vi "Vision_demo.vi"() -> ()   [LabVIEW 2011]
doc: "Use this template to build a standard state machine design pattern. Each state executes code and determines which state to transition to. Contrast this design pattern with the User Interface Event Handler pattern, in which code executes in response to user actions. Contrast this design pattern also with the Queued Message Handler pattern, in which each message handling code can queue zero or more new messages."
uses:
  StateMachineStates 1.ctl
  <vilib>/DAQmx/write.llb/DAQmx Write (Digital Bool 1Line 1Point).vi
  <vilib>/DAQmx/read.llb/DAQmx Read (Digital Bool 1Line 1Point).vi
  <vilib>/DAQmx/read.llb/DAQmx Read (Counter U32 1Chan 1Samp).vi
  <vilib>/DAQmx/miscellaneous.llb/DAQmx Fill In Error Info.vi
  <vilib>/DAQmx/create/channels.llb/DAQmx Create Channel (CI-Count Edges).vi
  <vilib>/DAQmx/read.llb/DAQmx Read (Counter DBL 1Chan 1Samp).vi
  <vilib>/DAQmx/create/channels.llb/DAQmx Create Channel (CI-Pulse Width).vi
panel:
  out "Set 4":bool[](array[boolean])
  out "Set 3":bool[](array[boolean])
  out "Set 2":bool[](array[boolean])
  out "Set 1":bool[](array[boolean])
  out "Photon time (ms)":dbl format="%.2f"
  in  "Interval (ms)":u32
  out "Repetition":dbl
  in  "Repetitions":dbl=1.0
  out "WP time (ms)":u32
  out "VISA Handle out":refnum<visa-resource-name>="ASRL5::INSTR"
  out "Initializing":bool
  out "Trial mode":T1(ring)
  in  "Frequency of LED trials\nfor Mixed mode":dbl=30.0
  out "Bright trial\nrequested":bool
  out "Observer Ready":bool
  in  "Bright/mixed mode \nLED voltage (V)":dbl=2.6 min=-3.0 max=4.0 format="%.2f"
  in  "Manual voltage (V)":dbl=2.6 format="%.2p"
  in  "GPIB address":string="15"
  in  "Period (ms)":i64=20
  in  "Pulse length (ms)":dbl=50.0
  out "L/R WP":dbl format="%.2f"
  in  "Manually \ninitialize":bool
  in  "COM for WPs":u8=5
  in  "L/R control method":enum16{"Liquid crystal", "Motorized waveplate"}(ring)=enum."Motorized waveplate"
  out "Blocked trial #":i32
  in  "Manual photon #":i32
  out "Photon #":i32
  out "LED Voltage":dbl
  in  "Blocking requirements":cluster{"Value":dbl, " Number":i32}[](array[cluster])
  in  "Manual":bool
  in  "Path":path=path "C:/Users/Lab/Dropbox/Vision software/Data"
  out "Counts 2":u32
  out "Counts 1":u32
  in  "Delay for APDs (ms)":u32=25
  in  "Counter 2":tag="Dev1/ctr1"
  in  "Counter 1":tag="Dev1/ctr0"
  out "Trial #":i32
  in  "Mode":T2(ring)=enum."Mixed"
  in  "Audio":bool=TRUE
  in  "Self-paced":bool
  out "Stimulus":bool
  out "Location Set":bool
  out "Stimulus \nlocation":string
  out "Waiting":bool
  out "Observer Responded":bool
  out "Response \ntime (ms)":dbl
  out "Observer \nchoice":string
  out "Confidence":i32
  in  "stop":bool
  in  "Next Trial":bool
  in  "Create New File":bool
  out "Subject #":string
  # "Settings for Blocking\nand Mixed Mode"
  # "Instructions: Run VI. Enter blocking requirements, then press\nCreate New File. Initialize waveplates if necessary, and set\nhighlighted controls to desired values. Press Next Trial to begin."
  # "Researcher Interface"
  # "Trial Options"
  # "Counter Options\n(same for LED &\ndetector tests)"
  # "Trial Information"
  # "Enter pre-set blocking \nrequirements\nbefore creating a new file."
  # "Troubleshooting"
  # "Photon Options"
  # "LED Options"
  # "Waveplates"
  # "Status"
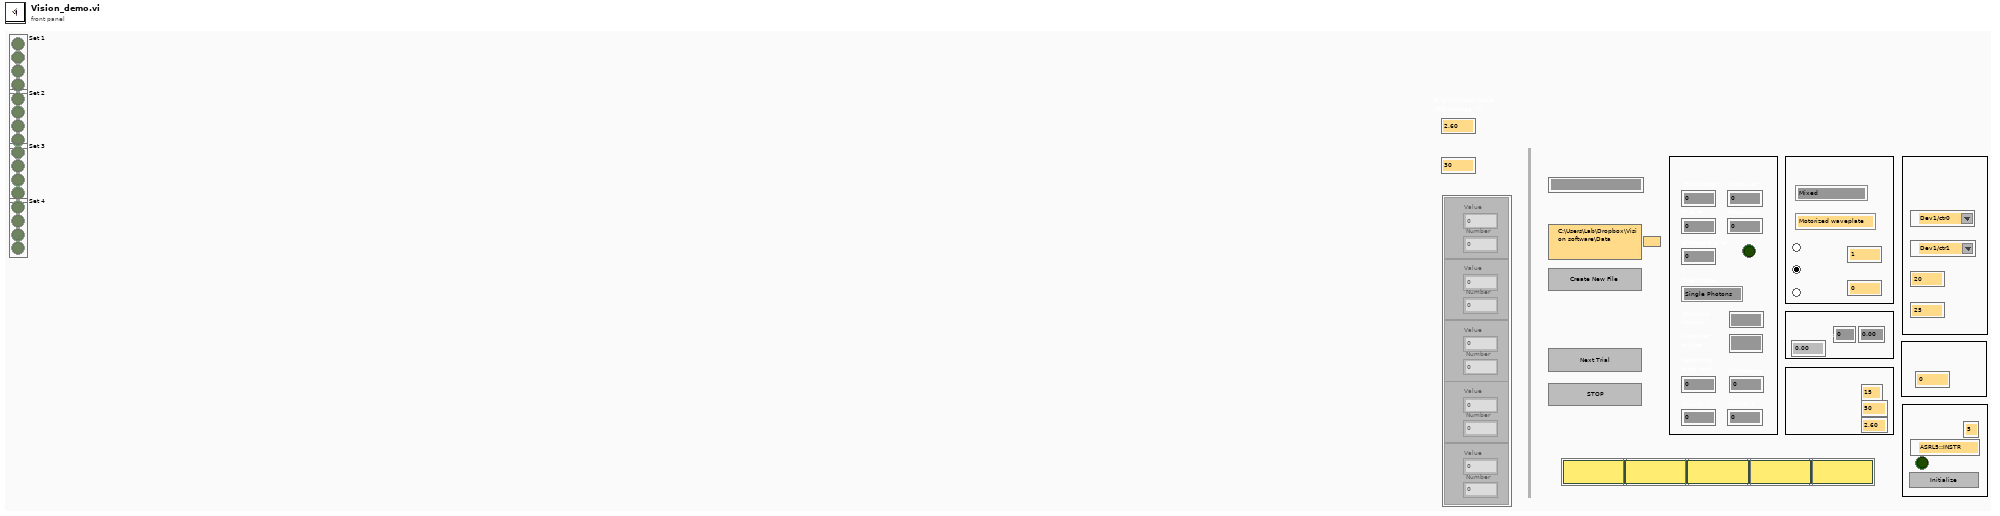
[diagram p1: front panel]
types:
  T1 = enum16{"Single Photons", "Detector Tests", "LED", "Mixed LED"}
  T2 = enum16{"Single Photons", "Detector Tests", "LED", "Mixed"}
  T3 = typedef "StateMachineStates 1.ctl" = enum16{"WaitResearcher", "SetWP", "SetLC", "WaitObserverReady", "Photons", "Detectors", "LED", "WaitObserverResponse", "CleanUp", "Stop"}
  T4 = enum16{"0", "1", "2", "3", "4", "5", "6", "7", "8", "9", "A", "B", "C", "D", "E", "F", "G", "H", "I", "J", "K", "L", "M", "N", "O", "P", "Q", "R", "S", "T", "U", "V", "W", "X", "Y", "Z", "F1", "F2", "F3", "F4", "F5", "F6", "F7", "F8", "F9", "F10", "F11", "F12", "F13", "F14", "F15", "ADD", "BACK", "BACKSLASH", "CAPITAL", "COMMA", "DECIMAL", "DELETE", "DIVIDE", "DOWN", "END", "EQUALS", "ESCAPE", "GRAVE (`)", "HOME", "INSERT", "LBRACKET", "LCONTROL", "LEFT", "L ALT", "LSHIFT", "LWIN", "MINUS", "MULTIPLY", "NEXT", "NUMLOCK", "NUMPAD_0", "NUMPAD_1", "NUMPAD_2", "NUMPAD_3", "NUMPAD_4", "NUMPAD_5", "NUMPAD_6", "NUMPAD_7", "NUMPAD_8", "NUMPAD_9", "PAUSE", "PERIOD", "PRIOR (PG UP)", "RBRACKET", "RCONTROL", "RETURN", "RIGHT", "R ALT", "RSHIFT", "RWIN", "SCROLL", "SEMICOLON", "SLASH", "SPACE", "SUBTRACT", "TAB", "UP", "ENTER (num pad)", "' (quote)"}
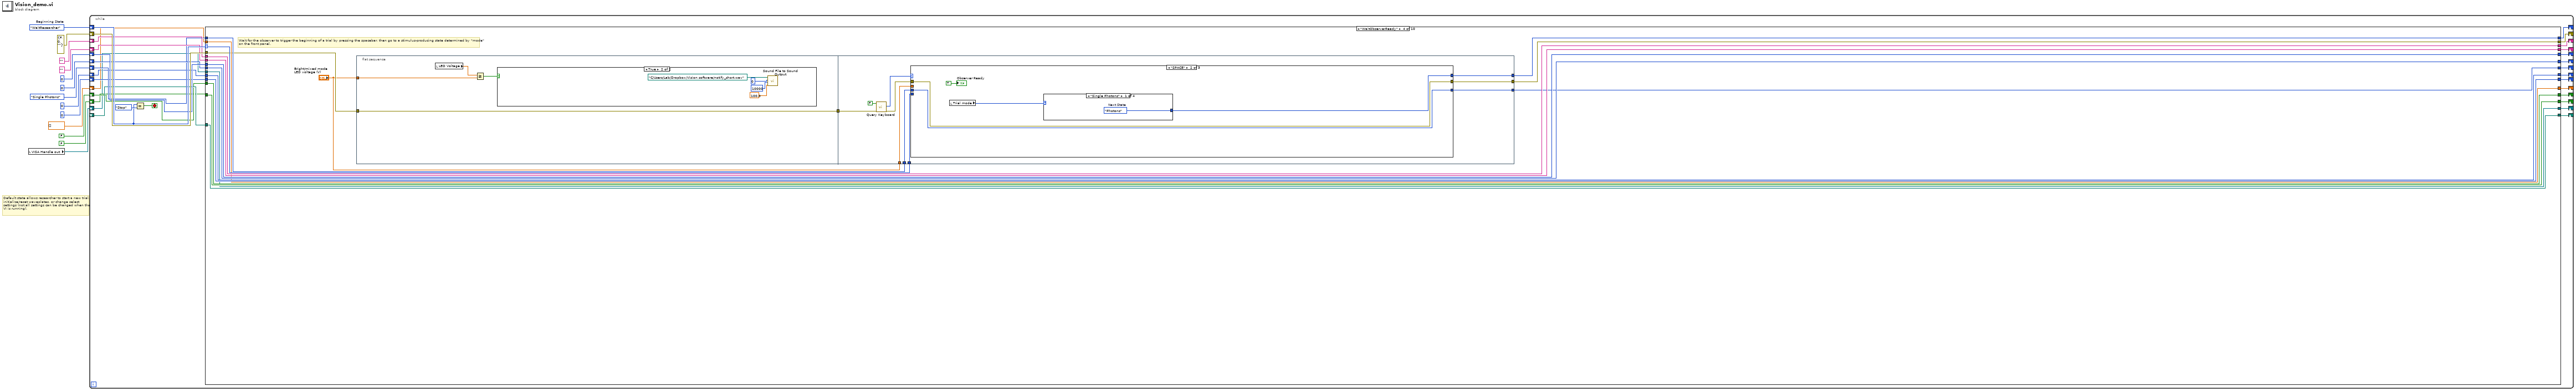
[diagram p0: block diagram]
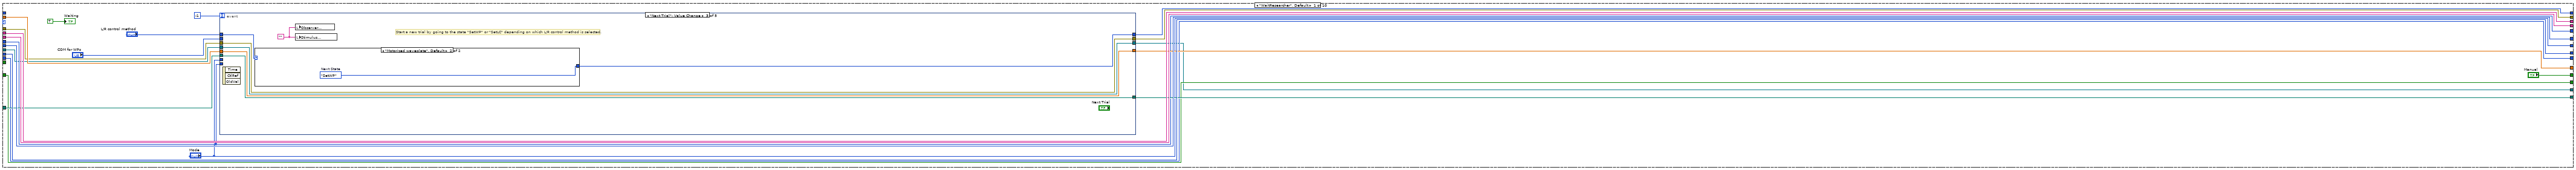
[diagram p2: hidden frame]
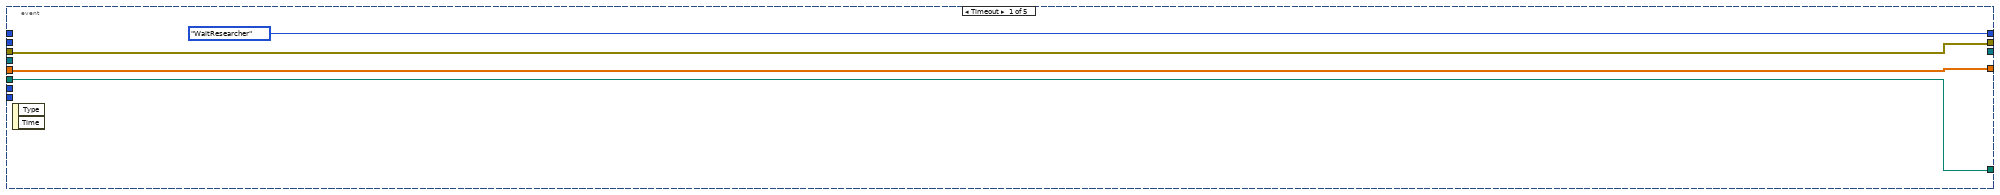
[diagram p3: hidden frame]
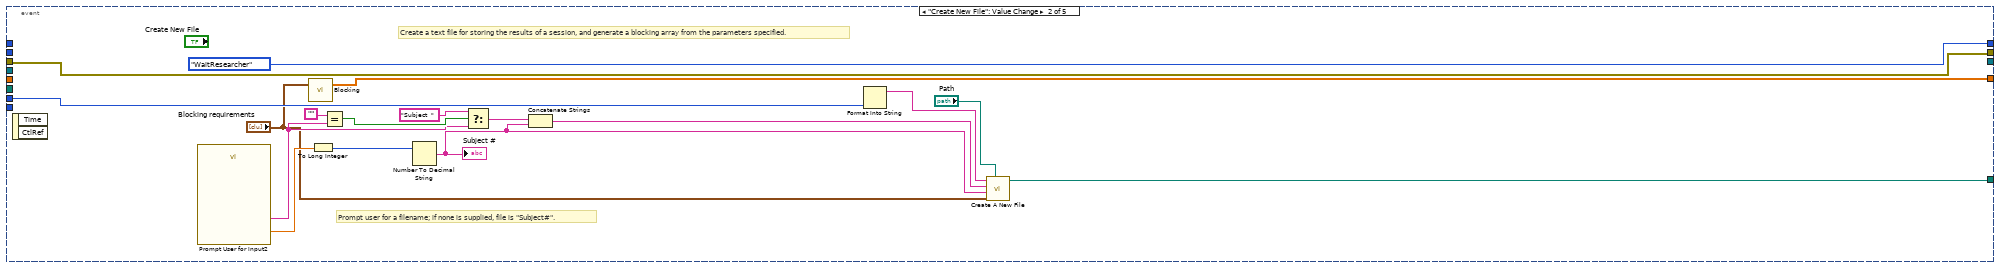
[diagram p4: hidden frame]
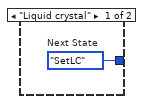
[diagram p5: hidden frame]
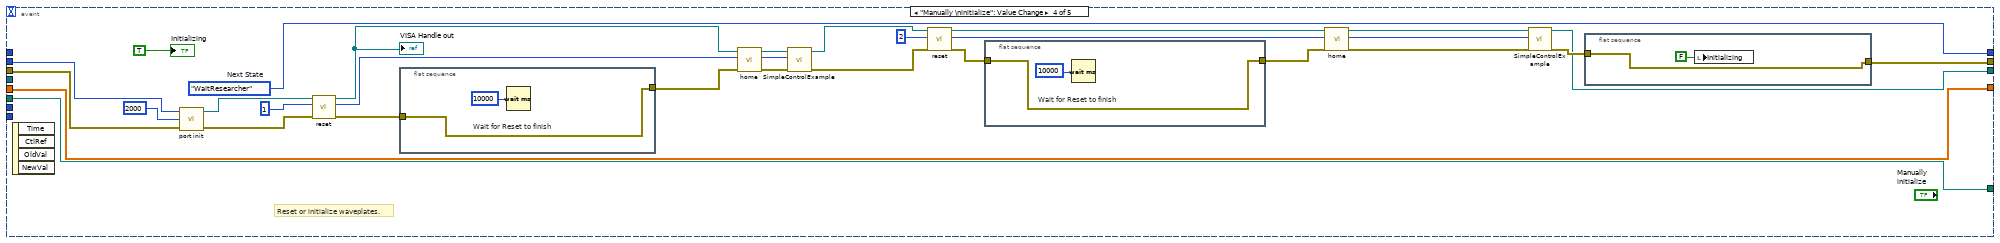
[diagram p6: hidden frame]
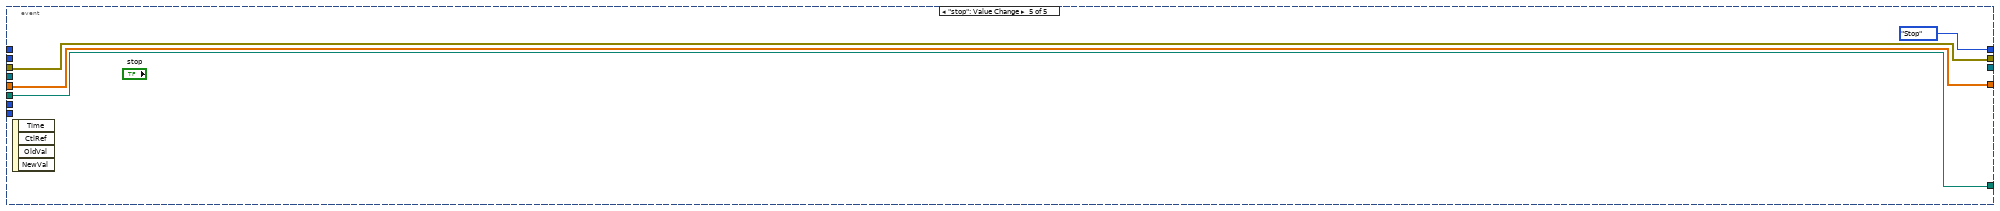
[diagram p7: hidden frame]
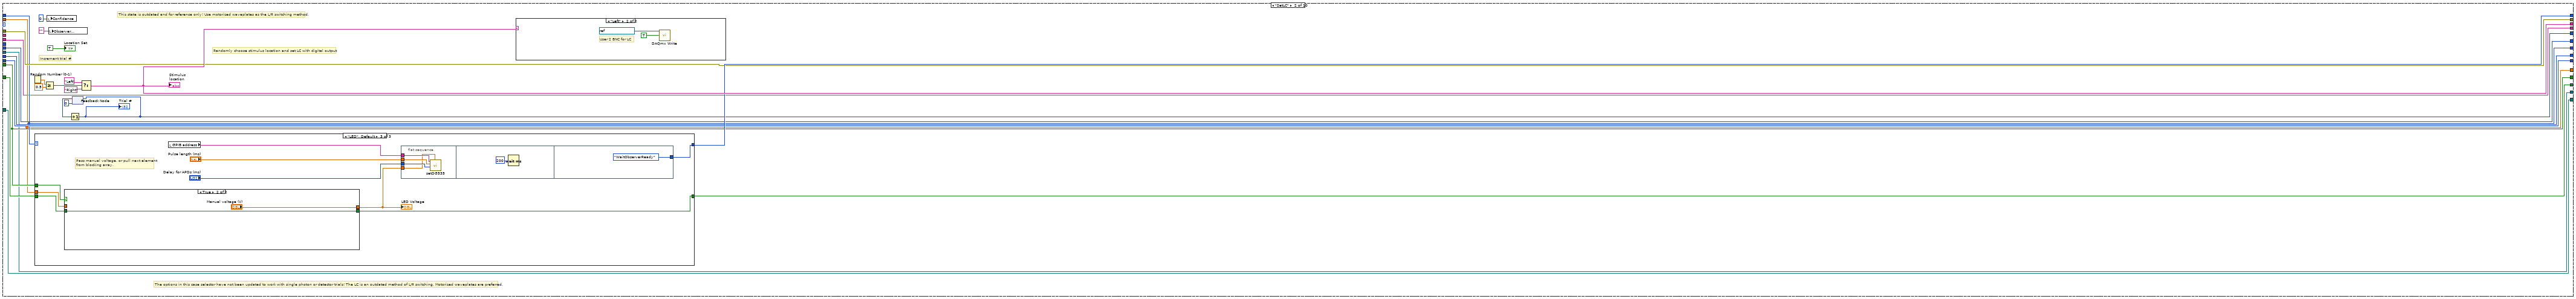
[diagram p8: hidden frame]
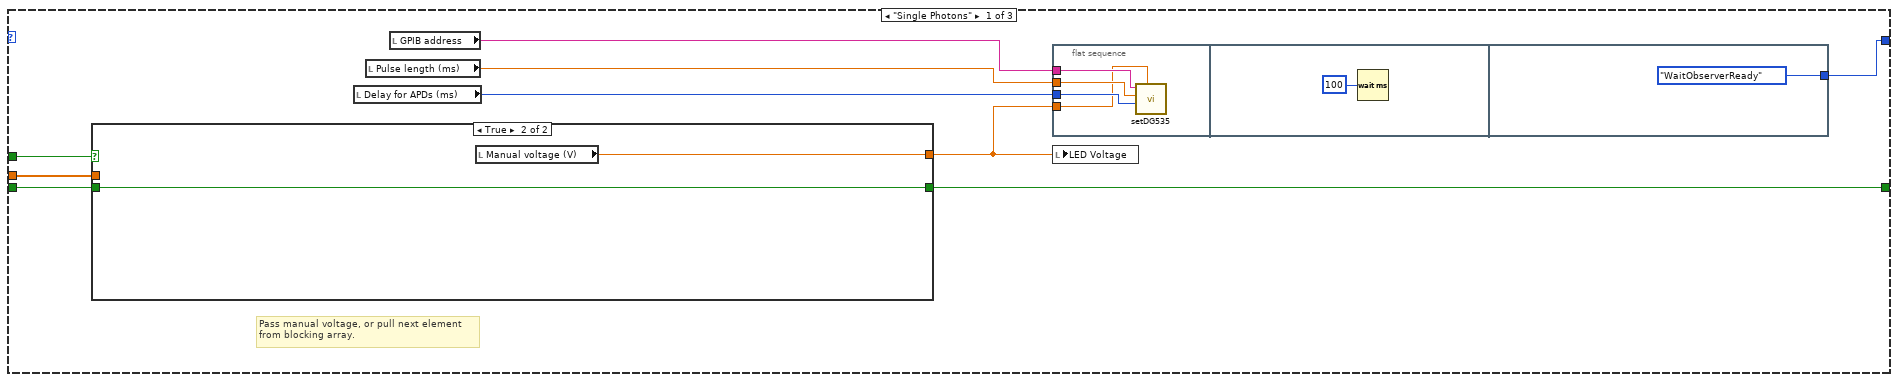
[diagram p9: hidden frame]
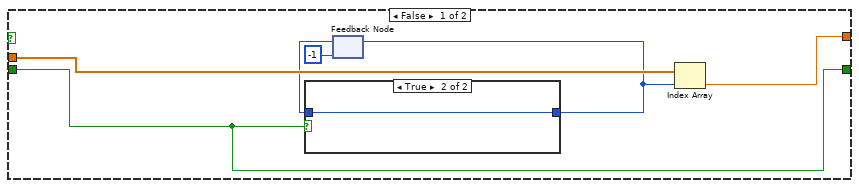
[diagram p10: hidden frame]
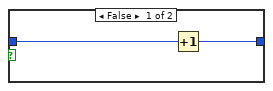
[diagram p11: hidden frame]
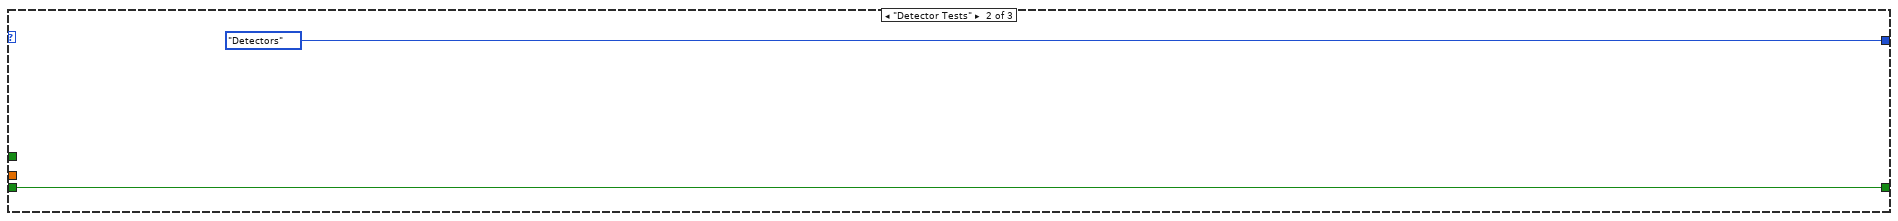
[diagram p12: hidden frame]
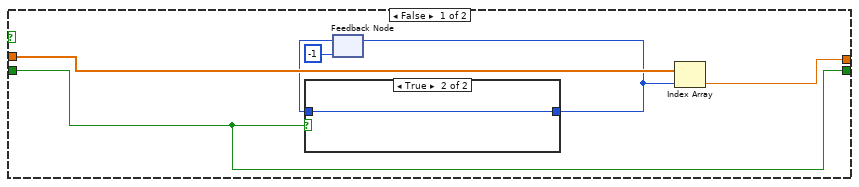
[diagram p13: hidden frame]
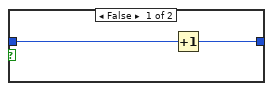
[diagram p14: hidden frame]
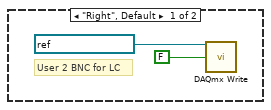
[diagram p15: hidden frame]
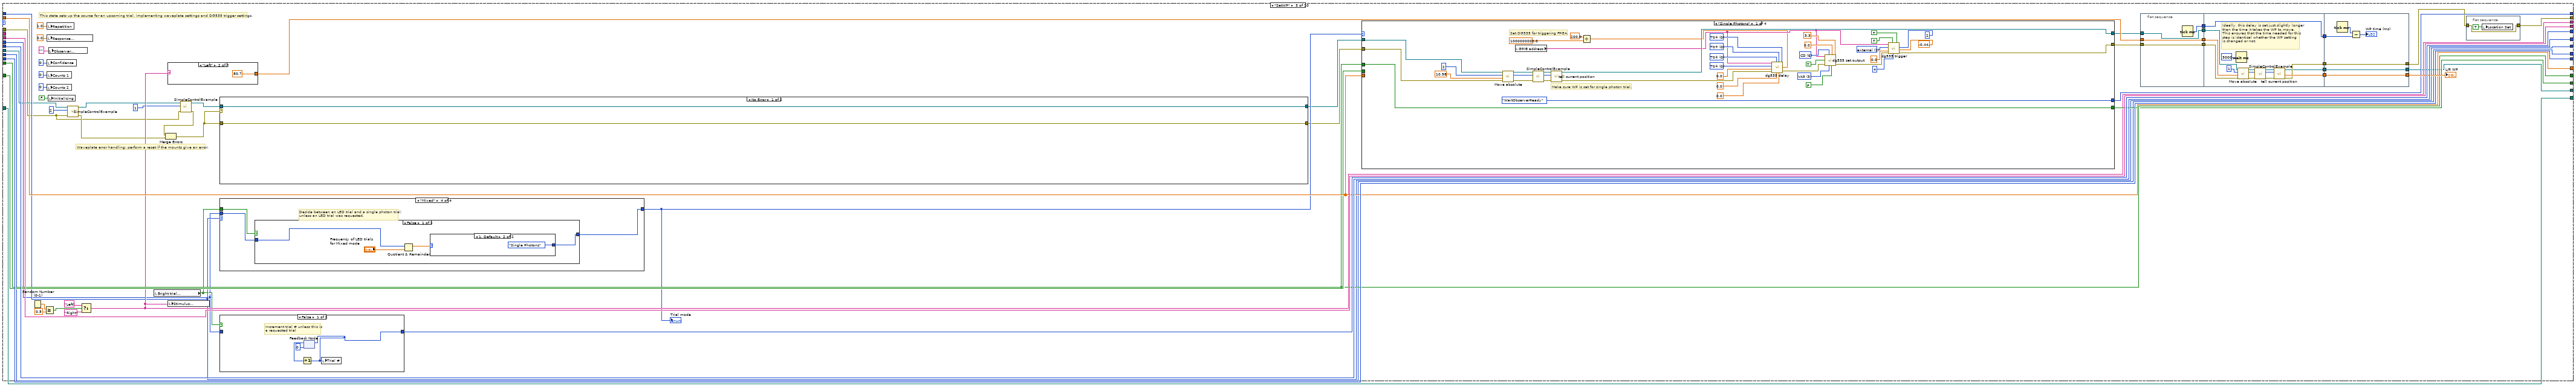
[diagram p16: hidden frame]
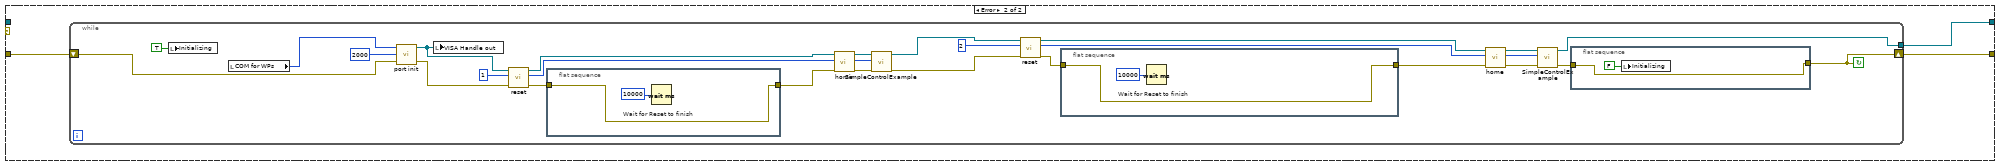
[diagram p17: hidden frame]
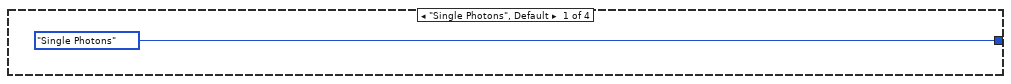
[diagram p19: hidden frame]
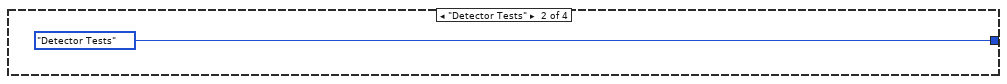
[diagram p20: hidden frame]
diagram:
  w13 = StateMachineStates_1."WaitResearcher"  # Beginning State
  # "Default state allows researcher to start a new trial,\ninitialize/reset waveplates, or change select\nsettings (not all settings can be changed when the\nVI is running)."
  n1 = local read "VISA Handle out"() -> (w1:refnum<visa-resource-name>)
  n2 = while {
    shift-right: [w40] -> _
    shift-left: w13 -> [w41]
    shift-right: [w19] -> _
    shift-left: errorcluster {"status"=FALSE, "code"=0, "source"=""} ("error out") -> [w39]
    shift-right: [w38] -> _
    shift-left: "" -> [w37]
    shift-right: [w36] -> _
    shift-left: "" ("Observer choice") -> [w35]
    shift-right: [w34] -> _
    shift-left: 0 -> [w33]
    shift-right: [w32] -> _
    shift-left: 0 ("Confidence") -> [w31]
    shift-right: [w30] -> _
    shift-left: T2."Single Photons" ("Mode") -> [w29]
    shift-right: [w28] -> _
    shift-left: u32 0 ("Counts 1") -> [w14]
    shift-right: [w27] -> _
    shift-left: u32 0 ("Counts 2") -> [w26]
    shift-right: [w25] -> _
    shift-left: _ -> [w24]
    shift-right: [w23] -> _
    shift-left: dbl[] [] ("Blocking array") -> [w22]
    shift-right: [w21] -> _
    shift-left: FALSE ("Manual") -> [w20]
    shift-right: [w18] -> _
    shift-left: FALSE ("Bright trial\nrequested") -> [w17]
    shift-right: [w16] -> _
    shift-left: w1 -> [w15]
    stop <- w43 stop-if-true
    n3 = Equal?(x=w41, y=StateMachineStates_1."Stop" ("States")) -> (x = y?=w43:bool)
    n4 = case shown="\"WaitObserverReady\"" w41 {
      selector: w41 -> [_ _ _ w521 _ _ _ _ _ _]
      tunnel: [w65 w154 w262 w522 StateMachineStates_1."WaitObserverResponse" ("Next State") w642 w832 w939 w1008 w1086] -> w40
      tunnel: [w50 w151 w261 w510 w601 w632 w818 w943 w991 w1091] -> w19
      tunnel: w39 -> [w51 w151 w220 w511 w587 w619 w834 w943 w985 w1090]
      tunnel: [w64 w155 w255 w525 w602 w645 w840 w945 w1004 w1102] -> w38
      tunnel: w37 -> [w64 _ _ w525 w602 w645 w840 w945 w1004 w1102]
      tunnel: [w63 w139 w272 w524 w605 w644 w813 w940 w1003 w1101] -> w36
      tunnel: w35 -> [w63 w139 w272 w524 w605 w644 _ _ w1003 w1101]
      tunnel: [w53 w145 w270 w523 w592 w635 w835 w944 w995 w1100] -> w34
      tunnel: w33 -> [w53 _ w236 w523 w592 w635 w835 w944 w995 w1100]
      tunnel: [w62 w152 w271 w520 w604 w643 w815 w938 w1007 w1099] -> w32
      tunnel: w31 -> [w62 w152 w271 w520 w604 w643 w815 _ w1007 w1099]
      tunnel: ["Mode" w144 w251 w518 w597 w641 w817 w937 w1002 w1098] -> w30
      tunnel: w29 -> [_ w144 w251 w517 w597 w641 w817 w937 w1002 w1098]
      tunnel: [w59 w148 w254 w516 w596 w640 w816 w936 w1000 w1097] -> w28
      tunnel: [w52 w147 w267 w515 w595 w639 w814 w935 w1001 w1096] -> w27
      tunnel: w14 -> [w59 w148 w254 w516 _ w640 _ w936 w1000 w1097]
      tunnel: w26 -> [w52 w147 w267 w515 _ w639 _ w935 w1001 w1096]
      tunnel: [w58 w146 w268 w514 w594 w638 w839 w934 w999 w1095] -> w25
      tunnel: w24 -> [w57 w146 w268 w514 w594 w638 w839 w934 w999 w1095]
      tunnel: [w56 w142 w266 w513 w593 w636 w836 w933 w997 w1094] -> w23
      tunnel: w22 -> [w55 w142 w266 w513 w593 w636 w836 w933 w997 w1094]
      tunnel: ["Manual" w143 w264 w512 w591 w637 w837 w932 w992 w1093] -> w21
      tunnel: w20 -> [_ w143 w264 w512 w591 w637 w837 w932 w989 w1093]
      tunnel: [w47 w140 w263 w508 w586 w633 w830 w931 w987 w1092] -> w18
      tunnel: w17 -> [w47 w141 w265 w508 w586 w633 w830 w931 _ w1092]
      tunnel: [w46 w136 w248 w507 w585 w634 w829 w930 w986 w1089] -> w16
      tunnel: w15 -> [w44 w136 w229 w507 w585 w634 w829 w930 w986 w1089]
      frame "WaitResearcher", Default {
        n5 = event shown="[2] \"Next Trial\": Value Change" {
          selector: _ -> [_ _ _ _ _]
          dyn-events: _ -> [_ _ _ _ _]
          timeout: -1 -> [_ _ _ _ _]
          tunnel: [StateMachineStates_1."WaitResearcher" ("Next State") StateMachineStates_1."WaitResearcher" ("Next State") w90 w125 StateMachineStates_1."Stop" ("Next State")] -> w65
          tunnel: "Mode" -> [_ w78 _ _ _]
          tunnel: [w69 w71 w92 w124 w134] -> w58
          tunnel: w57 -> [w69 _ w92 w124 w134]
          tunnel: [w68 w75 w91 w112 w133] -> w56
          tunnel: w55 -> [w68 _ w91 w112 w133]
          tunnel: w53 -> [_ _ _ _ _]
          tunnel: w51 -> [w67 w70 w88 w113 w132]
          tunnel: [w67 w70 w88 w102 w132] -> w50
          tunnel: "L/R control method" -> [_ _ w89 _ _]
          tunnel: "COM for WPs" -> [_ _ _ w100 _]
          tunnel: [_ _ w87 w98 _] -> w46
          tunnel: w44 -> [_ _ w87 _ _]
          event Timeout {
            n6 = event-data() -> ()  [unwired: 1 in, 2 out]
          }
          event "Create New File": Value Change {
            # "Create a text file for storing the results of a session, and generate a blocking array from the parameters specified."
            # "Prompt user for a filename; if none is supplied, file is \"Subject#\"."
            n7 = event-data() -> ()  [unwired: 1 in, 2 out]
            n8 = call "Prompt User for Input2"() -> ("Subject #"=w84:dbl, "Filename"=w81:string)  [unwired: 16 in, 2 out]
            n9 = call "Blocking.vi"("Blocking requirements"="Blocking requirements") -> ("Blocking array"=w75:dbl[])  [unwired: 2 in]
            n10 = To Long Integer(number=w84) -> (32bit integer=w85:i32)
            n11 = Equal?(x="", y=w81) -> (x = y?=w82:bool)
            n12 = Number To Decimal String(number=w85) -> (decimal integer string=w79:string)  [unwired: 1 in]
            "Subject #" <- w79
            n13 = Select(t="Subject  ", s=w82, f=w81) -> (s? t:f=w76:string)
            n14 = Concatenate Strings(w76, w79) -> (w72:string)
            n15 = Format Into String(w78) -> (resulting string=w77:string)  [unwired: 3 in, 1 out]
            n16 = call "Create A New File.vi"("Path in"="Path", "Blocking requirements"="Blocking requirements", "Subject #"=w79, "Filename"=w72, "Mode"=w77) -> ("Path out"=w71:path)  [unwired: 6 in]
          }
          event "Next Trial": Value Change {
            w93 = ""
            # "Start a new trial by going to the state \"SetWP\" or \"SetLC\" depending on which L/R control method is selected."
            n17 = event-data() -> ()  [unwired: 1 in, 3 out]
            n18 = case shown="\"Motorized waveplate\", Default" w89 {
              tunnel: [w94 w95] -> w90
              frame "Liquid crystal" {
                w94 = StateMachineStates_1."SetLC"  # Next State
              }
              frame "Motorized waveplate", Default {
                w95 = StateMachineStates_1."SetWP"  # Next State
              }
            }
            n19 = local write "Observer \nchoice"(w93) -> ()
            n20 = local write "Stimulus \nlocation"(w93) -> ()
          }
          event "Manually \ninitialize": Value Change {
            w125 = StateMachineStates_1."WaitResearcher"  # Next State
            # "Reset or initialize waveplates."
            n21 = event-data() -> ()  [unwired: 1 in, 4 out]
            n22 = call "port init.vi"("error in"=w113, "Timeout (300 ms)"=u32 2000, "SerialPort (1)"=w100) -> ("error out"=w120:errorcluster, "Visa Handle"=w119:refnum<visa-resource-name>)  [unwired: 1 in]
            n23 = call "reset.vi"("error in"=w120, "Axis in"=1, "VISA Handle in"=w119) -> ("error out"=w117:errorcluster, "Axis out"=w118:i32, "VISA Handle out"=w96:refnum<visa-resource-name>)  [unwired: 3 in, 1 out]
            "VISA Handle out" <- w96
            n24 = flat-sequence {
              tunnel: [w130] -> w116
              tunnel: w117 -> [w130]
              frame #0 {
                # "Wait for Reset to finish"
                n25 = Wait (ms)(milliseconds to wait=u32 10000) -> ()  [unwired: 1 out]
              }
            }
            n26 = call "home.vi"("error in"=w116, "Axis in"=w118, "VISA Handle in"=w96) -> ("error out"=w122:errorcluster, "Axis out"=w121:i32, "VISA Handle out"=w123:refnum<visa-resource-name>)  [unwired: 3 in, 1 out]
            n27 = call "SimpleControlExample.vi"("error in"=w122, "Axis in"=w121, "VISA Handle in"=w123) -> ("error out"=w101:errorcluster, "VISA Handle out"=w99:refnum<visa-resource-name>)  [unwired: 3 in, 2 out]
            n28 = call "reset.vi"("error in"=w101, "Axis in"=2, "VISA Handle in"=w99) -> ("error out"=w107:errorcluster, "Axis out"=w108:i32, "VISA Handle out"=w104:refnum<visa-resource-name>)  [unwired: 3 in, 1 out]
            n29 = flat-sequence {
              tunnel: [w128] -> w106
              tunnel: w107 -> [w128]
              frame #0 {
                # "Wait for Reset to finish"
                n30 = Wait (ms)(milliseconds to wait=u32 10000) -> ()  [unwired: 1 out]
              }
            }
            n31 = call "home.vi"("error in"=w106, "Axis in"=w108, "VISA Handle in"=w104) -> ("error out"=w110:errorcluster, "Axis out"=w109:i32, "VISA Handle out"=w111:refnum<visa-resource-name>)  [unwired: 3 in, 1 out]
            n32 = call "SimpleControlExample.vi"("error in"=w110, "Axis in"=w109, "VISA Handle in"=w111) -> ("error out"=w103:errorcluster, "VISA Handle out"=w98:refnum<visa-resource-name>)  [unwired: 3 in, 2 out]
            n33 = flat-sequence {
              tunnel: w103 -> [w127]
              tunnel: [w127] -> w102
              frame #0 {
                n34 = local write "Initializing"(FALSE ("Initializing waveplates")) -> ()
              }
            }
            "Initializing" <- TRUE ("Initializing waveplates")
          }
          event "stop": Value Change {
            n35 = event-data() -> ()  [unwired: 1 in, 4 out]
          }
        }
        "Waiting" <- TRUE ("Waiting")
      }
      frame "SetLC" {
        # "This state is outdated and for reference only! Use motorized waveplates as the L/R switching method."
        # "The options in this case selector have not been updated to work with single photon or detector trials! The LC is an outdated method of L/R switching. Motorized waveplates are preferred."
        # "Randomly choose stimulus location and set LC with digital output"
        # "Increment trial #"
        n36 = Random Number (0-1)() -> (number: 0 to 1=w160:dbl)
        n37 = case shown="\"LED\", Default" w144 {
          tunnel: [w166 StateMachineStates_1."Detectors" ("Next State") w191] -> w154
          tunnel: w143 -> [w169 _ w197]
          tunnel: w142 -> [w168 _ w196]
          tunnel: w141 -> [w165 w187 w190]
          tunnel: [w164 w187 w189] -> w140
          frame "Single Photons" {
            # "Pass manual voltage, or pull next element\nfrom blocking array."
            n38 = case shown="True" w169 {
              tunnel: [w180 w185] -> w161
              tunnel: w168 -> [w181 _]
              tunnel: w165 -> [w176 w186]
              tunnel: [w176 w186] -> w164
              frame False {
                n39 = feedback #1(-1 ("x+1")) -> (w179:i32)
                n40 = case shown="True" w176 {
                  tunnel: w179 -> [w183 w184]
                  tunnel: [w182 w184] -> w177
                  frame False {
                    n41 = Increment(x=w183) -> (x+1=w182:i32)
                  }
                  frame True {
                  }
                }
                n42 = feedback-in #1(w177) -> ()
                n43 = Index Array(array=w181, index=w177) -> (element=w180:dbl)
              }
              frame True {
                n44 = local read "Manual voltage (V)"() -> (w185:dbl)
              }
            }
            n45 = local read "Delay for APDs (ms)"() -> (w163:u32)
            n46 = local read "Pulse length (ms)"() -> (w162:dbl)
            n47 = local read "GPIB address"() -> (w167:string)
            n48 = flat-sequence {
              tunnel: w163 -> [w173]
              tunnel: w167 -> [w172]
              tunnel: w162 -> [w171]
              tunnel: w161 -> [w170]
              tunnel: [StateMachineStates_1."WaitObserverReady" ("Next State")] -> w166
              frame #0 {
                n49 = call "setDG535.vi"("amplitude"=w170, "Delay (ms)"=w173, "Pulse length (ms)"=w171, "GPIB address"=w172) -> ()  [unwired: 7 in, 1 out]
              }
              frame #1 {
                n50 = Wait (ms)(milliseconds to wait=u32 100) -> ()  [unwired: 1 out]
              }
              frame #2 {
              }
            }
            n51 = local write "LED Voltage"(w161) -> ()
          }
          frame "Detector Tests" {
          }
          frame "LED", Default {
            # "Pass manual voltage, or pull next element\nfrom blocking array."
            n52 = case shown="True" w197 {
              tunnel: [w208 "Manual voltage (V)"] -> w192
              tunnel: w196 -> [w209 _]
              tunnel: w190 -> [w204 w213]
              tunnel: [w204 w213] -> w189
              frame False {
                n53 = feedback #2(-1 ("x+1")) -> (w207:i32)
                n54 = case shown="True" w204 {
                  tunnel: w207 -> [w211 w212]
                  tunnel: [w210 w212] -> w205
                  frame False {
                    n55 = Increment(x=w211) -> (x+1=w210:i32)
                  }
                  frame True {
                  }
                }
                n56 = feedback-in #2(w205) -> ()
                n57 = Index Array(array=w209, index=w205) -> (element=w208:dbl)
              }
              frame True {
              }
            }
            "LED Voltage" <- w192
            n58 = local read "GPIB address"() -> (w194:string)
            n59 = flat-sequence {
              tunnel: "Delay for APDs (ms)" -> [w201]
              tunnel: w194 -> [w200]
              tunnel: "Pulse length (ms)" -> [w199]
              tunnel: w192 -> [w198]
              tunnel: [StateMachineStates_1."WaitObserverReady" ("Next State")] -> w191
              frame #0 {
                n60 = call "setDG535.vi"("amplitude"=w198, "Delay (ms)"=w201, "Pulse length (ms)"=w199, "GPIB address"=w200) -> ()  [unwired: 7 in, 1 out]
              }
              frame #1 {
                n61 = Wait (ms)(milliseconds to wait=u32 200) -> ()  [unwired: 1 out]
              }
              frame #2 {
              }
            }
          }
        }
        n62 = Greater Or Equal?(x=w160, y=0.5) -> (x >= y?=w158:bool)
        n63 = local write "Confidence"(0 ("Confidence")) -> ()
        n64 = local write "Observer \nchoice"("" ("Observer choice")) -> ()
        n65 = feedback #3(0 ("x+1")) -> (w150:i32)
        n66 = Increment(x=w150) -> (x+1=w145:i32)
        "Trial #" <- w145
        n67 = feedback-in #3(w145) -> ()
        n68 = Select(t="Left", s=w158, f="Right") -> (s? t:f=w155:string)
        "Stimulus \nlocation" <- w155
        n69 = case shown="\"Left\"" w155 {
          frame "Right", Default {
            # "User 2 BNC for LC"
            n70 = call-poly <vilib>:"DAQmx Write.vi"("task/channels in"=refnum<k21> "LC_Controller", "data"=FALSE) -> ()  [unwired: 11 in, 3 out]
          }
          frame "Left" {
            # "User 2 BNC for LC"
            n71 = call-poly <vilib>:"DAQmx Write.vi"("task/channels in"=refnum<k21> "LC_Controller", "data"=TRUE) -> ()  [unwired: 11 in, 3 out]
          }
        }
        "Location Set" <- TRUE ("LC Set")
      }
      frame "SetWP" {
        # "Waveplate error handling: perform a reset if the mounts give an error."
        # "This state sets up the source for an upcoming trial, implementing waveplate settings and DG535 trigger settings."
        n72 = Random Number (0-1)() -> (number: 0 to 1=w256:dbl)
        n73 = Greater Or Equal?(x=w256, y=0.5) -> (x >= y?=w258:bool)
        n74 = local write "Repetition"(1.0 ("Repitition #")) -> ()
        n75 = local write "Response \ntime (ms)"(0.0 ("Response \ntime (ms)")) -> ()
        n76 = local write "Confidence"(0 ("Confidence")) -> ()
        n77 = local write "Counts 1"(u32 0 ("Counts 1")) -> ()
        n78 = local write "Counts 2"(u32 0 ("Counts 2")) -> ()
        n79 = local write "Initializing"(FALSE ("Initializing waveplates")) -> ()
        n80 = local write "Observer \nchoice"("" ("Observer \nchoice")) -> ()
        n81 = call "SimpleControlExample.vi"("error in"=w220, "Axis in"=2, "VISA Handle in"=w229) -> ("error out"=w221:errorcluster, "VISA Handle out"=w227:refnum<visa-resource-name>)  [unwired: 3 in, 2 out]
        n82 = Select(t="Left", s=w258, f="Right") -> (s? t:f=w255:string)
        n83 = local read "Bright trial\nrequested"() -> (w237:bool)
        n84 = case shown="\"Left\"" w255 {
          tunnel: [35.7 ("New target position (units)") 80.7 ("New target position (units)")] -> w252
          frame "Right", Default {
          }
          frame "Left" {
          }
        }
        n85 = local write "Stimulus \nlocation"(w255) -> ()
        n86 = call "SimpleControlExample.vi"("error in"=w220, "Axis in"=1, "VISA Handle in"=w227) -> ("error out"=w222:errorcluster, "VISA Handle out"=w225:refnum<visa-resource-name>)  [unwired: 3 in, 2 out]
        n87 = Merge Errors(w222, w221) -> (w219:errorcluster)
        n88 = case shown="No Error" w219 {
          tunnel: w219 -> [w274 w277]
          tunnel: [w274 w275] -> w223
          tunnel: [w273 w276] -> w224
          tunnel: w225 -> [w273 _]
          frame No Error {
          }
          frame Error {
            n89 = while {
              tunnel: [w280] -> w276
              shift-right: [w278] -> w275
              shift-left: w277 -> [w283]
              stop <- w278 continue-if-true
              n90 = local write "Initializing"(TRUE ("Initializing waveplates")) -> ()
              n91 = local read "COM for WPs"() -> (w282:u8)
              n92 = call "port init.vi"("error in"=w283, "Timeout (300 ms)"=u32 2000, "SerialPort (1)"=w282) -> ("error out"=w301:errorcluster, "Visa Handle"=w281:refnum<visa-resource-name>)  [unwired: 1 in]
              n93 = local write "VISA Handle out"(w281) -> ()
              n94 = call "reset.vi"("error in"=w301, "Axis in"=1, "VISA Handle in"=w281) -> ("error out"=w299:errorcluster, "Axis out"=w300:i32, "VISA Handle out"=w284:refnum<visa-resource-name>)  [unwired: 3 in, 1 out]
              n95 = flat-sequence {
                tunnel: [w309] -> w298
                tunnel: w299 -> [w309]
                frame #0 {
                  # "Wait for Reset to finish"
                  n96 = Wait (ms)(milliseconds to wait=u32 10000) -> ()  [unwired: 1 out]
                }
              }
              n97 = call "home.vi"("error in"=w298, "Axis in"=w300, "VISA Handle in"=w284) -> ("error out"=w303:errorcluster, "Axis out"=w302:i32, "VISA Handle out"=w304:refnum<visa-resource-name>)  [unwired: 3 in, 1 out]
              n98 = call "SimpleControlExample.vi"("error in"=w303, "Axis in"=w302, "VISA Handle in"=w304) -> ("error out"=w286:errorcluster, "VISA Handle out"=w285:refnum<visa-resource-name>)  [unwired: 3 in, 2 out]
              n99 = call "reset.vi"("error in"=w286, "Axis in"=2, "VISA Handle in"=w285) -> ("error out"=w291:errorcluster, "Axis out"=w292:i32, "VISA Handle out"=w288:refnum<visa-resource-name>)  [unwired: 3 in, 1 out]
              n100 = flat-sequence {
                tunnel: [w307] -> w290
                tunnel: w291 -> [w307]
                frame #0 {
                  # "Wait for Reset to finish"
                  n101 = Wait (ms)(milliseconds to wait=u32 10000) -> ()  [unwired: 1 out]
                }
              }
              n102 = call "home.vi"("error in"=w290, "Axis in"=w292, "VISA Handle in"=w288) -> ("error out"=w294:errorcluster, "Axis out"=w293:i32, "VISA Handle out"=w295:refnum<visa-resource-name>)  [unwired: 3 in, 1 out]
              n103 = call "SimpleControlExample.vi"("error in"=w294, "Axis in"=w293, "VISA Handle in"=w295) -> ("error out"=w287:errorcluster, "VISA Handle out"=w280:refnum<visa-resource-name>)  [unwired: 3 in, 2 out]
              n104 = flat-sequence {
                tunnel: w287 -> [w306]
                tunnel: [w306] -> w278
                frame #0 {
                  n105 = local write "Initializing"(FALSE ("Initializing waveplates")) -> ()
                }
              }
            }
          }
        }
        n106 = case shown="\"Mixed\"" w251 {
          tunnel: [T1."Single Photons" ("Mode") T1."Detector Tests" ("Mode") T1."LED" ("Mode") w319] -> w250
          tunnel: w236 -> [_ _ _ w320]
          tunnel: w237 -> [_ _ _ w318]
          frame "Single Photons", Default {
          }
          frame "Detector Tests" {
          }
          frame "LED" {
          }
          frame "Mixed" {
            # "Decide between an LED trial and a single photon trial,\nunless an LED trial was requested."
            n107 = case shown="False" w318 {
              tunnel: w320 -> [w324 _]
              tunnel: [w321 T1."Mixed LED" ("Mode")] -> w319
              frame False {
                n108 = Quotient & Remainder(x=w324, y="Frequency of LED trials\nfor Mixed mode") -> (x-y*floor(x/y)=w322:dbl)  [unwired: 1 out]
                n109 = case shown="1, Default" w322 {
                  tunnel: [T1."Mixed LED" ("Mode") T1."Single Photons" ("Mode")] -> w321
                  frame 0 {
                  }
                  frame 1, Default {
                  }
                }
              }
              frame True {
              }
            }
          }
        }
        "Trial mode" <- w250
        n110 = case shown="False" w237 {
          tunnel: [w311 w314] -> w270
          tunnel: w236 -> [_ w314]
          frame False {
            # "Increment trial # unless this is\na requested trial"
            n111 = feedback #4(0 ("x+1")) -> (w313:i32)
            n112 = Increment(x=w313) -> (x+1=w311:i32)
            n113 = feedback-in #4(w311) -> ()
            n114 = local write "Trial #"(w311) -> ()
          }
          frame True {
          }
        }
        n115 = case shown="\"Single Photons\"" w250 {
          tunnel: [StateMachineStates_1."WaitObserverReady" ("Next State") StateMachineStates_1."Detectors" ("Next State") w456 w496] -> w262
          tunnel: w264 -> [w397 _ w459 _]
          tunnel: w266 -> [_ _ w458 _]
          tunnel: w265 -> [_ w437 w455 w482]
          tunnel: [w397 w437 w454 w482] -> w263
          tunnel: w223 -> [w388 w429 w443 w486]
          tunnel: [w358 w398 w442 w477] -> w246
          tunnel: w224 -> [w357 w427 w440 w484]
          tunnel: [w386 w426 w439 w483] -> w247
          frame "Single Photons" {
            w374 = u32 1 items=["internal", "external", "single shot", "burst", "line"] ("trigger")
            w376 = 3 items=["TTL", "NIM", "ECL", "VAR"] ("mode")
            w378 = u16 6 items=["T0", "A", "B", "AB", "C", "D", "CD"] ("output")
            w381 = u32 0 items=["T0+", "A+", "B+", "C+"] ("D=")
            w382 = u32 0 items=["T0+", "A+", "B+", "D+"] ("C=")
            w383 = u32 0 items=["T0+", "A+", "C+", "D+"] ("B=")
            w384 = u32 0 items=["T0+", "B+", "C+", "D+"] ("A=")
            # "Set DG535 for triggering FPGA."
            # "Make sure WP is set for single photon trial."
            n116 = call <instrlib>:"Move absolute.vi"("error in"=w388, "New target position (units)"=10.98, "Axis in"=2, "VISA Handle in"=w357) -> ("error out"=w390:errorcluster, "Axis out"=w391:i32, "VISA Handle out"=w392:refnum<visa-resource-name>)  [unwired: 2 in, 1 out]
            n117 = local read "GPIB address"() -> (w366:string)
            n118 = call "SimpleControlExample.vi"("error in"=w390, "Axis in"=w391, "VISA Handle in"=w392) -> ("error out"=w393:errorcluster, "Axis out"=w394:i32, "VISA Handle out"=w395:refnum<visa-resource-name>)  [unwired: 3 in, 1 out]
            n119 = call "tell current position.vi"("error in"=w393, "Axis in"=w394, "VISA Handle in"=w395) -> ("error out"=w359:errorcluster, "VISA Handle out"=w386:refnum<visa-resource-name>)  [unwired: 2 in, 3 out]
            n120 = Divide(x=200.0 ("D"), y=1000000000.0) -> (x/y=w360:dbl)
            n121 = call "dg535 delay.vi"("C"=0.0, "D"=w360, "D="=w381, "C="=w382, "B"=0.0 ("C"), "error in"=w359, "A"=0.0 ("D"), "B="=w383, "A="=w384, "GPIB address"=w366) -> ("error out"=w380:errorcluster)
            n122 = call "dg535 set output.vi"("GPIB address"=w366, "output"=w378, "set"=TRUE, "error in"=w380, "mode"=w376, "offset"=0.0, "amplitude"=3.3, "load"=FALSE) -> ("error out"=w367:errorcluster)  [unwired: 1 in]
            n123 = call "dg535 trigger.vi"("external trigger level"=sgl -0.45, "burst count"=2, "trigger slope"=TRUE, "burst period"=4, "input impedance"=TRUE, "error in"=w367, "internal/burst trigger rate"=0.0, "trigger"=w374, "GPIB address"=w366) -> ("error out"=w358:errorcluster)
          }
          frame "Detector Tests" {
            w414 = u32 1 items=["internal", "external", "single shot", "burst", "line"] ("trigger")
            w416 = 3 items=["TTL", "NIM", "ECL", "VAR"] ("mode")
            w418 = u16 6 items=["T0", "A", "B", "AB", "C", "D", "CD"] ("output")
            w421 = u32 0 items=["T0+", "A+", "B+", "C+"] ("D=")
            w422 = u32 0 items=["T0+", "A+", "B+", "D+"] ("C=")
            w423 = u32 0 items=["T0+", "A+", "C+", "D+"] ("B=")
            w424 = u32 0 items=["T0+", "B+", "C+", "D+"] ("A=")
            # "Set DG535 for triggering FPGA."
            # "Make sure WP is set for single photon trial."
            n124 = local read "GPIB address"() -> (w406:string)
            n125 = Divide(x=200.0 ("D"), y=1000000000.0) -> (x/y=w400:dbl)
            n126 = call <instrlib>:"Move absolute.vi"("error in"=w429, "New target position (units)"=10.98, "Axis in"=2, "VISA Handle in"=w427) -> ("error out"=w431:errorcluster, "Axis out"=w432:i32, "VISA Handle out"=w433:refnum<visa-resource-name>)  [unwired: 2 in, 1 out]
            n127 = call "SimpleControlExample.vi"("error in"=w431, "Axis in"=w432, "VISA Handle in"=w433) -> ("error out"=w434:errorcluster, "Axis out"=w435:i32, "VISA Handle out"=w436:refnum<visa-resource-name>)  [unwired: 3 in, 1 out]
            n128 = call "tell current position.vi"("error in"=w434, "Axis in"=w435, "VISA Handle in"=w436) -> ("error out"=w399:errorcluster, "VISA Handle out"=w426:refnum<visa-resource-name>)  [unwired: 2 in, 3 out]
            n129 = call "dg535 delay.vi"("C"=0.0, "D"=w400, "D="=w421, "C="=w422, "B"=0.0 ("C"), "error in"=w399, "A"=0.0 ("D"), "B="=w423, "A="=w424, "GPIB address"=w406) -> ("error out"=w420:errorcluster)
            n130 = call "dg535 set output.vi"("GPIB address"=w406, "output"=w418, "set"=TRUE, "error in"=w420, "mode"=w416, "offset"=0.0, "amplitude"=3.3, "load"=FALSE) -> ("error out"=w407:errorcluster)  [unwired: 1 in]
            n131 = call "dg535 trigger.vi"("external trigger level"=sgl -0.45, "burst count"=2, "trigger slope"=TRUE, "burst period"=4, "input impedance"=TRUE, "error in"=w407, "internal/burst trigger rate"=0.0, "trigger"=w414, "GPIB address"=w406) -> ("error out"=w398:errorcluster)
          }
          frame "LED", Default {
            # "Make sure WP is set for LED trial."
            # "Set relevent parameters on DG535 for LED flash."
            # "Pass manual voltage, or pull next element\nfrom blocking array."
            n132 = case shown="False" w459 {
              tunnel: [w470 w475] -> w453
              tunnel: w458 -> [w471 _]
              tunnel: w455 -> [w466 w476]
              tunnel: [w466 w476] -> w454
              frame False {
                n133 = feedback #5(-1 ("x+1")) -> (w469:i32)
                n134 = case shown="True" w466 {
                  tunnel: w469 -> [w473 w474]
                  tunnel: [w472 w474] -> w467
                  frame False {
                    n135 = Increment(x=w473) -> (x+1=w472:i32)
                  }
                  frame True {
                  }
                }
                n136 = feedback-in #5(w467) -> ()
                n137 = Index Array(array=w471, index=w467) -> (element=w470:dbl)
              }
              frame True {
                n138 = local read "Manual voltage (V)"() -> (w475:dbl)
              }
            }
            n139 = local read "Delay for APDs (ms)"() -> (w451:u32)
            n140 = local read "Pulse length (ms)"() -> (w452:dbl)
            n141 = local read "GPIB address"() -> (w457:string)
            n142 = call <instrlib>:"Move absolute.vi"("error in"=w443, "New target position (units)"=55.98, "Axis in"=2, "VISA Handle in"=w440) -> ("error out"=w445:errorcluster, "Axis out"=w446:i32, "VISA Handle out"=w447:refnum<visa-resource-name>)  [unwired: 2 in, 1 out]
            n143 = local write "LED Voltage"(w453) -> ()
            n144 = flat-sequence {
              tunnel: w451 -> [w463]
              tunnel: w457 -> [w462]
              tunnel: w452 -> [w461]
              tunnel: w453 -> [w460]
              tunnel: [StateMachineStates_1."WaitObserverReady" ("Next State")] -> w456
              frame #0 {
                n145 = call "setDG535.vi"("amplitude"=w460, "Delay (ms)"=w463, "Pulse length (ms)"=w461, "GPIB address"=w462) -> ()  [unwired: 7 in, 1 out]
              }
              frame #1 {
                n146 = Wait (ms)(milliseconds to wait=u32 100) -> ()  [unwired: 1 out]
              }
              frame #2 {
              }
            }
            n147 = call "SimpleControlExample.vi"("error in"=w445, "Axis in"=w446, "VISA Handle in"=w447) -> ("error out"=w448:errorcluster, "Axis out"=w449:i32, "VISA Handle out"=w450:refnum<visa-resource-name>)  [unwired: 3 in, 1 out]
            n148 = call "tell current position.vi"("error in"=w448, "Axis in"=w449, "VISA Handle in"=w450) -> ("error out"=w442:errorcluster, "VISA Handle out"=w439:refnum<visa-resource-name>)  [unwired: 2 in, 3 out]
          }
          frame "Mixed LED" {
            # "Make sure WP is set for LED trial."
            # "Set relevent parameters on DG535 for LED flash."
            n149 = local read "Delay for APDs (ms)"() -> (w494:u32)
            n150 = call <instrlib>:"Move absolute.vi"("error in"=w486, "New target position (units)"=55.98, "Axis in"=2, "VISA Handle in"=w484) -> ("error out"=w488:errorcluster, "Axis out"=w489:i32, "VISA Handle out"=w490:refnum<visa-resource-name>)  [unwired: 2 in, 1 out]
            n151 = local read "Pulse length (ms)"() -> (w495:dbl)
            n152 = local read "GPIB address"() -> (w497:string)
            n153 = call "SimpleControlExample.vi"("error in"=w488, "Axis in"=w489, "VISA Handle in"=w490) -> ("error out"=w491:errorcluster, "Axis out"=w492:i32, "VISA Handle out"=w493:refnum<visa-resource-name>)  [unwired: 3 in, 1 out]
            n154 = local read "Bright/mixed mode \nLED voltage (V)"() -> (w481:dbl)
            n155 = call "tell current position.vi"("error in"=w491, "Axis in"=w492, "VISA Handle in"=w493) -> ("error out"=w480:errorcluster, "VISA Handle out"=w483:refnum<visa-resource-name>)  [unwired: 2 in, 3 out]
            n156 = local write "LED Voltage"(w481) -> ()
            n157 = flat-sequence {
              tunnel: w494 -> [w502]
              tunnel: w497 -> [w501]
              tunnel: w495 -> [w500]
              tunnel: w481 -> [w499]
              tunnel: w480 -> [w498]
              tunnel: [w498] -> w478
              tunnel: [w503] -> w479
              tunnel: w478 -> [w503]
              tunnel: [StateMachineStates_1."WaitObserverReady" ("Next State")] -> w496
              tunnel: [w505] -> w477
              tunnel: w479 -> [w505]
              frame #0 {
                n158 = call "setDG535.vi"("amplitude"=w499, "Delay (ms)"=w502, "Pulse length (ms)"=w500, "GPIB address"=w501) -> ()  [unwired: 7 in, 1 out]
              }
              frame #1 {
                n159 = Wait (ms)(milliseconds to wait=u32 100) -> ()  [unwired: 1 out]
              }
              frame #2 {
              }
            }
          }
        }
        n160 = flat-sequence {
          tunnel: w247 -> [w329]
          tunnel: w252 -> [w330]
          tunnel: w246 -> [w331]
          tunnel: [w331] -> w245
          tunnel: [w330] -> w244
          tunnel: [w329] -> w243
          tunnel: [w328] -> w238
          tunnel: w245 -> [w338]
          tunnel: w244 -> [w335]
          tunnel: w243 -> [w334]
          tunnel: [w339] -> w242
          tunnel: [w337] -> w241
          tunnel: [w333] -> w240
          tunnel: [w332] -> w239
          tunnel: w238 -> [w332]
          tunnel: [w350] -> w248
          tunnel: [w351] -> w253
          tunnel: [w352] -> w269
          tunnel: w242 -> [w352]
          tunnel: w241 -> [w351]
          tunnel: w240 -> [w350]
          tunnel: w239 -> [w349]
          frame #0 {
            n161 = Tick Count (ms)() -> (millisecond timer value=w328:u32)
          }
          frame #1 {
            # "Ideally, this delay is set just slightly longer\nthan the time it takes the WP to move.\nThis ensures that the time needed for this\nstep is identical whether the WP setting\nis changed or not."
            n162 = Wait (ms)(milliseconds to wait=u32 3000) -> ()  [unwired: 1 out]
            n163 = call <instrlib>:"Move absolute.vi"("error in"=w338, "New target position (units)"=w335, "Axis in"=1, "VISA Handle in"=w334) -> ("error out"=w341:errorcluster, "Axis out"=w342:i32, "VISA Handle out"=w343:refnum<visa-resource-name>)  [unwired: 2 in, 1 out]
            n164 = call "SimpleControlExample.vi"("error in"=w341, "Axis in"=w342, "VISA Handle in"=w343) -> ("error out"=w344:errorcluster, "Axis out"=w345:i32, "VISA Handle out"=w346:refnum<visa-resource-name>)  [unwired: 3 in, 1 out]
            n165 = call "tell current position.vi"("error in"=w344, "Axis in"=w345, "VISA Handle in"=w346) -> ("error out"=w337:errorcluster, "Current position (units)"=w339:dbl, "VISA Handle out"=w333:refnum<visa-resource-name>)  [unwired: 2 in, 2 out]
          }
          frame #2 {
            n166 = Tick Count (ms)() -> (millisecond timer value=w348:u32)
            n167 = Subtract(x=w348, y=w349) -> (x-y=→"WP time (ms)":u32)
          }
        }
        n168 = flat-sequence {
          tunnel: w253 -> [w355]
          tunnel: [w355] -> w261
          frame #0 {
            n169 = local write "Location Set"(TRUE ("Location Set")) -> ()
          }
        }
        "L/R WP" <- w269
      }
      frame "WaitObserverReady" {
        # "Wait for the observer to trigger the beginning of a trial by pressing the spacebar, then go to a stimulus-producing state determined by \"mode\"\non the front panel."
        n170 = flat-sequence {
          tunnel: [w526] -> w519
          tunnel: w511 -> [w526]
          tunnel: "Bright/mixed mode \nLED voltage (V)" -> [w529]
          tunnel: w521 -> [w542]
          tunnel: w519 -> [w540]
          tunnel: w517 -> [w535]
          tunnel: "Bright/mixed mode \nLED voltage (V)" -> [w534]
          tunnel: [w536] -> w510
          tunnel: [w543] -> w522
          tunnel: [w539] -> w518
          frame #0 {
            n171 = local read "LED Voltage"() -> (w528:dbl)
            n172 = Greater Or Equal?(x=w528, y=w529) -> (x >= y?=w527:bool)
            n173 = case shown="True" w527 {
              frame False {
                n174 = call <vilib>:"Beep.vi"() -> ()  [unwired: 12 in]
              }
              frame True {
                n175 = call "Sound File to Sound Output.vi"("Volume"=100.0, "Number of Samples/Iteration"=10000, "Device ID"=u32 0, "File Path"=path "C:/Users/Lab/Dropbox/Vision software/notify_short.wav") -> ()
              }
            }
          }
          frame #1 {
            n176 = call "Query Keyboard.vi"("error in (no error)"=w540, "Stop?"=FALSE) -> ("error out"=w537:errorcluster, "element"=w541:T4)  [unwired: 8 in]
            n177 = case shown="\"SPACE\"" w541 {
              tunnel: [StateMachineStates_1."WaitObserverReady" ("Next State") w551 w558] -> w543
              tunnel: w542 -> [_ _ _]
              tunnel: [w545 w550 w556] -> w539
              tunnel: w535 -> [w545 w550 w556]
              tunnel: w537 -> [w544 w548 w560]
              tunnel: [w544 w548 w559] -> w536
              tunnel: w534 -> [_ _ w557]
              frame "1", Default {
              }
              frame "SPACE" {
                n178 = local read "Trial mode"() -> (w547:T1)
                n179 = case shown="\"Single Photons\"" w547 {
                  tunnel: [w552 w553 w554 w555] -> w551
                  frame "Single Photons" {
                    w552 = StateMachineStates_1."Photons"  # Next State
                  }
                  frame "Detector Tests" {
                    w553 = StateMachineStates_1."Detectors"  # Next State
                  }
                  frame "LED", Default {
                    w554 = StateMachineStates_1."LED"  # Next State
                  }
                  frame "Mixed LED" {
                    w555 = StateMachineStates_1."LED"  # Next State
                  }
                }
                "Observer Ready" <- TRUE ("Observer Ready")
              }
              frame "NUMPAD_0" {
                n180 = case shown="\"Mixed\"" w556 {
                  tunnel: w560 -> [w561 w563 w568 w583]
                  tunnel: [w561 w563 w567 w583] -> w559
                  tunnel: [StateMachineStates_1."WaitObserverReady" ("Next State") StateMachineStates_1."WaitObserverReady" ("Next State") w566 StateMachineStates_1."SetWP" ("Next State")] -> w558
                  tunnel: w557 -> [_ _ w565 _]
                  frame "Single Photons", Default {
                  }
                  frame "Detector Tests" {
                  }
                  frame "LED" {
                    n181 = flat-sequence {
                      tunnel: w568 -> [w573]
                      tunnel: [w572] -> w570
                      tunnel: w565 -> [w571]
                      tunnel: w570 -> [w578]
                      tunnel: [w578] -> w569
                      tunnel: [w581] -> w567
                      tunnel: w569 -> [w581]
                      tunnel: [StateMachineStates_1."WaitObserverReady" ("Next State")] -> w566
                      frame #0 {
                        n182 = local write "LED Voltage"(w571) -> ()
                        n183 = local read "Delay for APDs (ms)"() -> (w575:u32)
                        n184 = local read "Pulse length (ms)"() -> (w574:dbl)
                        n185 = local read "GPIB address"() -> (w576:string)
                        n186 = call "setDG535.vi"("amplitude"=w571, "error in"=w573, "Delay (ms)"=w575, "Pulse length (ms)"=w574, "GPIB address"=w576) -> ("error out"=w572:errorcluster)  [unwired: 6 in]
                      }
                      frame #1 {
                        n187 = Wait (ms)(milliseconds to wait=u32 100) -> ()  [unwired: 1 out]
                      }
                      frame #2 {
                        "Bright trial\nrequested" <- TRUE ("Requested")
                      }
                    }
                  }
                  frame "Mixed" {
                    n188 = local write "Bright trial\nrequested"(TRUE ("Bright trial\nrequested")) -> ()
                  }
                }
              }
            }
          }
        }
      }
      frame "LED" {
        # "Flash LED while reading out counts from two single-photon detectors."
        n189 = local write "Photon #"(0.0 ("Photon #")) -> ()
        n190 = call "flashLED_DG535andcount.vi"("error in"=w587, "GPIB address"="GPIB address", "Period"="Period (ms)", "Counter 2"="Counter 2", "Counter 1"="Counter 1") -> ("Counts 2"=w595:u32, "Counts 1"=w596:u32, "error out"=w600:errorcluster)  [unwired: 4 in]
        "Counts 1" <- w596
        "Counts 2" <- w595
        n191 = flat-sequence {
          tunnel: w600 -> [w606]
          tunnel: [w606] -> w601
          frame #0 {
            "Stimulus" <- TRUE ("Stimulus")
          }
        }
      }
      frame "Photons" {
        w618 = 10.0  # timeout
        w622 = 10280 items=["Rising"=10280, "Falling"=10171] ("Starting Edge")
        # "If specified # of repetitions has been reached, go to\nWaitObserverResponse. If not, repeat Photons and increment\nRepetition #, pausing for Interval time before proceeding."
        # "Pass manual photon # or pull next element from\nblocking array. If there are multiple repetitions,\ndo this only on repetition 1; for the others, use the same\nphoton #."
        n192 = local read "Repetition"() -> (w628:dbl)
        n193 = Greater Or Equal?(x=w628, y="Repetitions") -> (x >= y?=w631:bool)
        n194 = Less Or Equal?(x=w628, y=1.0 ("x")) -> (x <= y?=w629:bool)
        n195 = case shown="True" w629 {
          tunnel: w637 -> [_ w789]
          tunnel: w636 -> [_ w788]
          tunnel: w635 -> [_ w787]
          tunnel: [w784 w786] -> w609
          tunnel: w633 -> [_ w785]
          frame False {
            n196 = local read "Photon #"() -> (w784:i32)
          }
          frame True {
            n197 = case shown="True" w789 {
              tunnel: [w796 "Manual photon #"] -> w786
              tunnel: w788 -> [w791 _]
              tunnel: w787 -> [_ _]
              tunnel: w785 -> [w792 _]
              frame False {
                n198 = feedback #6(-1 ("x+1")) -> (w795:i32)
                n199 = case shown="False" w792 {
                  tunnel: w795 -> [w798 w799]
                  tunnel: [w797 w799] -> w793
                  frame False {
                    n200 = Increment(x=w798) -> (x+1=w797:i32)
                  }
                  frame True {
                  }
                }
                n201 = feedback-in #6(w793) -> ()
                n202 = Index Array(array=w791, index=w793) -> (element=w790:dbl)
                n203 = To Long Integer(number=w790) -> (32bit integer=w796:i32)
              }
              frame True {
              }
            }
          }
        }
        "Photon #" <- w609
        n204 = call-poly <vilib>:"DAQmx Create Virtual Channel.vi"("maximum value"=0.5 ("Maximum Value (sec)"), "minimum value"=0.1 ("Minimum Value (sec)"), "counter"=tag "Dev1/ctr3" ("Physical Channel"), "error in"=w619, "starting edge"=w622) -> ("task out"=w623:refnum<k21>, "error out"=w610:errorcluster)  [unwired: 9 in]
        n205 = call-poly <vilib>:"DAQmx Read.vi"("task/channels in"=w623, "timeout"=w618) -> ("task out"=w621:refnum<k21>, "data"=w616:dbl, "error out"=w620:errorcluster)  [unwired: 11 in]
        n206 = call <vilib>:"DAQmx Clear Task.vi"("task in"=w621, "error in"=w620) -> ()  [unwired: 13 in, 1 out]
        n207 = Multiply(x=w616, y=1000.0) -> (x*y=→"Photon time (ms)":dbl)
        n208 = flat-sequence {
          tunnel: w610 -> [w647]
          tunnel: w609 -> [w650]
          tunnel: [w650] -> w614
          tunnel: [w646] -> w613
          tunnel: [w651] -> w612
          tunnel: w614 -> [w658]
          tunnel: w613 -> [w655]
          tunnel: w612 -> [w759]
          tunnel: [w758] -> w611
          tunnel: [w767] -> w608
          tunnel: w611 -> [w773]
          frame #0 {
            # "Reset load bit\nbefore transferring\ndata."
            n209 = call-poly <vilib>:"DAQmx Write.vi"("task/channels in"=refnum<k21> "BIT5", "data"=FALSE, "error in"=w647) -> ("error out"=w646:errorcluster)  [unwired: 10 in, 2 out]
          }
          frame #1 {
            # "P0.0 tells FPGA program \nto start."
            # "Convert number to a 16-bit\nunsigned integer."
            # "Transfer target count to FPGA as 4 sets of 4 bits."
            n210 = Number To Boolean Array(number=w658) -> (Boolean array=w656:bool[])
            n211 = for {
              N: 4 -> [_]
              tunnel: w656 -> [w662]
              tunnel: w655 -> [w664]
              tunnel: [w659] -> w652
              i -> [w665]
              n212 = Increment(x=w665) -> (x+1=w663:i32)
              n213 = flat-sequence {
                tunnel: w664 -> [w669]
                tunnel: w663 -> [w668]
                tunnel: w662 -> [w667]
                tunnel: [w666] -> w661
                tunnel: w661 -> [w751]
                tunnel: [w750] -> w660
                tunnel: w660 -> [w755]
                tunnel: [w754] -> w659
                frame #0 {
                  # "Transfer 4 bits of data: 1:4 on the first iteration, 5:8 on the\nsecond, and so on."
                  n214 = case shown="1, Default" w668 {
                    tunnel: w667 -> [w677 w697 w717 w737]
                    tunnel: w669 -> [w676 w696 w716 w736]
                    tunnel: [w675 w695 w715 w735] -> w666
                    frame 1, Default {
                      n215 = Index Array(array=w677, index=0) -> (element=w674:bool)
                      n216 = Index Array(array=w677, index=1) -> (element=w673:bool)
                      n217 = Index Array(array=w677, index=2) -> (element=w672:bool)
                      n218 = Index Array(array=w677, index=3) -> (element=w671:bool)
                      n219 = Build Array(w674, w673, w672, w671) -> (→"Set 1":bool[])
                      n220 = call-poly <vilib>:"DAQmx Write.vi"("task/channels in"=refnum<k21> "BIT1", "data"=w674, "error in"=w676) -> ("error out"=w685:errorcluster)  [unwired: 10 in, 2 out]
                      n221 = call-poly <vilib>:"DAQmx Write.vi"("task/channels in"=refnum<k21> "BIT2", "data"=w673) -> ("error out"=w684:errorcluster)  [unwired: 11 in, 2 out]
                      n222 = call-poly <vilib>:"DAQmx Write.vi"("task/channels in"=refnum<k21> "BIT3", "data"=w672) -> ("error out"=w683:errorcluster)  [unwired: 11 in, 2 out]
                      n223 = call-poly <vilib>:"DAQmx Write.vi"("task/channels in"=refnum<k21> "BIT4", "data"=w671) -> ("error out"=w682:errorcluster)  [unwired: 11 in, 2 out]
                      n224 = Merge Errors(w685, w684, w683, w682) -> (w675:errorcluster)
                    }
                    frame 2 {
                      n225 = Index Array(array=w697, index=4) -> (element=w694:bool)
                      n226 = Index Array(array=w697, index=5) -> (element=w693:bool)
                      n227 = Index Array(array=w697, index=6) -> (element=w692:bool)
                      n228 = Index Array(array=w697, index=7) -> (element=w691:bool)
                      n229 = Build Array(w694, w693, w692, w691) -> (→"Set 2":bool[])
                      n230 = call-poly <vilib>:"DAQmx Write.vi"("task/channels in"=refnum<k21> "BIT1", "data"=w694, "error in"=w696) -> ("error out"=w705:errorcluster)  [unwired: 10 in, 2 out]
                      n231 = call-poly <vilib>:"DAQmx Write.vi"("task/channels in"=refnum<k21> "BIT2", "data"=w693) -> ("error out"=w704:errorcluster)  [unwired: 11 in, 2 out]
                      n232 = call-poly <vilib>:"DAQmx Write.vi"("task/channels in"=refnum<k21> "BIT3", "data"=w692) -> ("error out"=w703:errorcluster)  [unwired: 11 in, 2 out]
                      n233 = call-poly <vilib>:"DAQmx Write.vi"("task/channels in"=refnum<k21> "BIT4", "data"=w691) -> ("error out"=w702:errorcluster)  [unwired: 11 in, 2 out]
                      n234 = Merge Errors(w705, w704, w703, w702) -> (w695:errorcluster)
                    }
                    frame 3 {
                      n235 = Index Array(array=w717, index=8) -> (element=w714:bool)
                      n236 = Index Array(array=w717, index=9) -> (element=w713:bool)
                      n237 = Index Array(array=w717, index=10) -> (element=w712:bool)
                      n238 = Index Array(array=w717, index=11) -> (element=w711:bool)
                      n239 = Build Array(w714, w713, w712, w711) -> (→"Set 3":bool[])
                      n240 = call-poly <vilib>:"DAQmx Write.vi"("task/channels in"=refnum<k21> "BIT1", "data"=w714, "error in"=w716) -> ("error out"=w725:errorcluster)  [unwired: 10 in, 2 out]
                      n241 = call-poly <vilib>:"DAQmx Write.vi"("task/channels in"=refnum<k21> "BIT2", "data"=w713) -> ("error out"=w724:errorcluster)  [unwired: 11 in, 2 out]
                      n242 = call-poly <vilib>:"DAQmx Write.vi"("task/channels in"=refnum<k21> "BIT3", "data"=w712) -> ("error out"=w723:errorcluster)  [unwired: 11 in, 2 out]
                      n243 = call-poly <vilib>:"DAQmx Write.vi"("task/channels in"=refnum<k21> "BIT4", "data"=w711) -> ("error out"=w722:errorcluster)  [unwired: 11 in, 2 out]
                      n244 = Merge Errors(w725, w724, w723, w722) -> (w715:errorcluster)
                    }
                    frame 4 {
                      n245 = Index Array(array=w737, index=12) -> (element=w734:bool)
                      n246 = Index Array(array=w737, index=13) -> (element=w733:bool)
                      n247 = Index Array(array=w737, index=14) -> (element=w732:bool)
                      n248 = Index Array(array=w737, index=15) -> (element=w731:bool)
                      n249 = Build Array(w734, w733, w732, w731) -> (→"Set 4":bool[])
                      n250 = call-poly <vilib>:"DAQmx Write.vi"("task/channels in"=refnum<k21> "BIT1", "data"=w734, "error in"=w736) -> ("error out"=w745:errorcluster)  [unwired: 10 in, 2 out]
                      n251 = call-poly <vilib>:"DAQmx Write.vi"("task/channels in"=refnum<k21> "BIT2", "data"=w733) -> ("error out"=w744:errorcluster)  [unwired: 11 in, 2 out]
                      n252 = call-poly <vilib>:"DAQmx Write.vi"("task/channels in"=refnum<k21> "BIT3", "data"=w732) -> ("error out"=w743:errorcluster)  [unwired: 11 in, 2 out]
                      n253 = call-poly <vilib>:"DAQmx Write.vi"("task/channels in"=refnum<k21> "BIT4", "data"=w731) -> ("error out"=w742:errorcluster)  [unwired: 11 in, 2 out]
                      n254 = Merge Errors(w745, w744, w743, w742) -> (w735:errorcluster)
                    }
                  }
                }
                frame #1 {
                  # "Set the load bit to high\nso FPGA reads the data."
                  n255 = call-poly <vilib>:"DAQmx Write.vi"("task/channels in"=refnum<k21> "BIT5", "data"=TRUE, "error in"=w751) -> ("error out"=w750:errorcluster)  [unwired: 10 in, 2 out]
                }
                frame #2 {
                  # "Reset load bit to low\nto prepare for next 4 bits\nor to end transfer after the\n4th set."
                  n256 = call-poly <vilib>:"DAQmx Write.vi"("task/channels in"=refnum<k21> "BIT5", "data"=FALSE, "error in"=w755) -> ("error out"=w754:errorcluster)  [unwired: 10 in, 2 out]
                }
              }
            }
            n257 = call-poly <vilib>:"DAQmx Write.vi"("task/channels in"=refnum<k21> "LaserChannel", "data"=TRUE, "error in"=w652) -> ("error out"=w651:errorcluster)  [unwired: 10 in, 2 out]
          }
          frame #2 {
            # "P0.2 tells LabVIEW that the FPGA is finished counting."
            n258 = while {
              tunnel: w759 -> [w765]
              tunnel: [w764] -> w758
              stop <- w761 stop-if-true
              n259 = Wait Until Next ms Multiple(millisecond multiple=u32 100) -> ()  [unwired: 1 out]
              n260 = call-poly <vilib>:"DAQmx Read.vi"("task/channels in"=refnum<k21> "P02countSignal", "error in"=w765) -> ("data"=w762:bool, "error out"=w764:errorcluster)  [unwired: 11 in, 1 out]
              n261 = Equal?(x=TRUE, y=w762) -> (x = y?=w761:bool)
            }
          }
          frame #3 {
            # "Reset all bits to low."
            # "Reset the P0.0 signal to low."
            n262 = call-poly <vilib>:"DAQmx Write.vi"("task/channels in"=refnum<k21> "BIT2", "data"=FALSE) -> ("error out"=w780:errorcluster)  [unwired: 11 in, 2 out]
            n263 = call-poly <vilib>:"DAQmx Write.vi"("task/channels in"=refnum<k21> "BIT3", "data"=FALSE) -> ("error out"=w779:errorcluster)  [unwired: 11 in, 2 out]
            n264 = call-poly <vilib>:"DAQmx Write.vi"("task/channels in"=refnum<k21> "BIT4", "data"=FALSE) -> ("error out"=w778:errorcluster)  [unwired: 11 in, 2 out]
            n265 = call-poly <vilib>:"DAQmx Write.vi"("task/channels in"=refnum<k21> "LaserChannel", "data"=FALSE, "error in"=w773) -> ("error out"=w772:errorcluster)  [unwired: 10 in, 2 out]
            n266 = call-poly <vilib>:"DAQmx Write.vi"("task/channels in"=refnum<k21> "BIT1", "data"=FALSE, "error in"=w772) -> ("error out"=w781:errorcluster)  [unwired: 10 in, 2 out]
            n267 = Merge Errors(w781, w780, w779, w778) -> (w767:errorcluster)
          }
        }
        n268 = case shown="True" w631 {
          tunnel: [StateMachineStates_1."Photons" ("States") StateMachineStates_1."WaitObserverResponse" ("States")] -> w642
          tunnel: w608 -> [w804 w811]
          tunnel: [w804 w811] -> w632
          tunnel: w628 -> [w803 _]
          frame False {
            n269 = Increment(x=w803) -> (x+1=→"Repetition":dbl)
            n270 = Wait (ms)(milliseconds to wait="Interval (ms)") -> ()  [unwired: 1 out]
          }
          frame True {
            n271 = local write "Stimulus"(TRUE ("Counts Taken")) -> ()
            n272 = call "Sound File to Sound Output.vi"("Volume"=100.0, "Number of Samples/Iteration"=10000, "Device ID"=u32 0, "File Path"=path "C:/Users/Lab/Dropbox/Vision software/Speech Misrecognition.wav") -> ()
          }
        }
      }
      frame "Detectors" {
        # "This state is outdated and non-functional! Needs to be updated to work with new FPGA program. 5/29/14"
        n273 = case shown="False" w837 {
          tunnel: [w923 w929] -> w831
          tunnel: w836 -> [w928 _]
          tunnel: w835 -> [w927 _]
          frame False {
            n274 = Subtract(x=w927, y=1) -> (x-y=w925:i32)
            n275 = Index Array(array=w928, index=w925) -> (element=w924:dbl)
            n276 = To Long Integer(number=w924) -> (32bit integer=w923:i32)
          }
          frame True {
            n277 = local read "Manual photon #"() -> (w929:i32)
          }
        }
        n278 = local write "LED Voltage"(0.0 ("LED Voltage")) -> ()
        n279 = flat-sequence {
          tunnel: [w841] -> w833
          tunnel: w834 -> [w842]
          tunnel: w831 -> [w843]
          tunnel: w833 -> [w849]
          tunnel: [w848] -> w828
          tunnel: [w847] -> w827
          tunnel: [w846] -> w826
          tunnel: w828 -> [w865]
          tunnel: [w865] -> w825
          tunnel: [w862] -> w823
          tunnel: w827 -> [w862]
          tunnel: [w861] -> w821
          tunnel: w826 -> [w861]
          tunnel: w825 -> [w867]
          tunnel: [w866] -> w824
          tunnel: w823 -> [w869]
          tunnel: [w869] -> w822
          tunnel: w821 -> [w868]
          tunnel: [w868] -> w820
          tunnel: w824 -> [w896]
          tunnel: [w890] -> w813
          tunnel: [w903] -> w814
          tunnel: [w902] -> w816
          tunnel: w822 -> [w894]
          tunnel: w820 -> [w893]
          tunnel: [w895] -> w819
          tunnel: [w922] -> w832
          tunnel: [w920] -> w818
          tunnel: w819 -> [w920]
          frame #0 {
            n280 = call "NtoFPGA.vi"("error in"=w842, "number"=w843) -> ("error out"=w841:errorcluster)  [unwired: 3 in]
          }
          frame #1 {
            w856 = 10128 items=["Count Up"=10128, "Count Down"=10124, "Externally Controlled"=10326] ("Count Direction")
            w857 = 10280 items=["Rising"=10280, "Falling"=10171] ("Edge")
            w859 = 10128 items=["Count Up"=10128, "Count Down"=10124, "Externally Controlled"=10326] ("Count Direction")
            w860 = 10280 items=["Rising"=10280, "Falling"=10171] ("Edge")
            n281 = local read "Counter 2"() -> (w844:tag)
            n282 = local read "Counter 1"() -> (w845:tag)
            n283 = call-poly <vilib>:"DAQmx Create Virtual Channel.vi"("initial count"=u32 0 ("Initial Count"), "count direction"=w856, "edge"=w857, "counter"=w845, "error in"=w849) -> ("task out"=w854:refnum<k21>, "error out"=w851:errorcluster)  [unwired: 9 in]
            n284 = call-poly <vilib>:"DAQmx Create Virtual Channel.vi"("initial count"=u32 0 ("Initial Count"), "count direction"=w859, "edge"=w860, "counter"=w844, "error in"=w851) -> ("task out"=w853:refnum<k21>, "error out"=w852:errorcluster)  [unwired: 9 in]
            n285 = call <vilib>:"DAQmx Start Task.vi"("task/channels in"=w853, "error in"=w852) -> ("task out"=w846:refnum<k21>, "error out"=w850:errorcluster)  [unwired: 12 in]
            n286 = call <vilib>:"DAQmx Start Task.vi"("task/channels in"=w854, "error in"=w850) -> ("task out"=w847:refnum<k21>, "error out"=w848:errorcluster)  [unwired: 12 in]
          }
          frame #2 {
            # "User 1/P0.0 for Laser"
            n287 = call-poly <vilib>:"DAQmx Write.vi"("task/channels in"=refnum<k21> "LaserChannel", "data"=TRUE) -> ()  [unwired: 11 in, 3 out]
          }
          frame #3 {
            n288 = while {
              tunnel: w867 -> [w875]
              tunnel: [w874] -> w866
              stop <- w871 stop-if-true
              n289 = Wait Until Next ms Multiple(millisecond multiple=u32 100) -> ()  [unwired: 1 out]
              n290 = call-poly <vilib>:"DAQmx Read.vi"("task/channels in"=refnum<k21> "P02countSignal", "error in"=w875) -> ("data"=w872:bool, "error out"=w874:errorcluster)  [unwired: 11 in, 1 out]
              n291 = Equal?(x=TRUE, y=w872) -> (x = y?=w871:bool)
            }
          }
          frame #4 {
            # "Right"
            # "Left"
            n292 = call-poly <vilib>:"DAQmx Read.vi"("task/channels in"=w893, "error in"=w896) -> ("task out"=w898:refnum<k21>, "data"=w882:u32, "error out"=w897:errorcluster)  [unwired: 11 in]
            n293 = To Unsigned Long Integer(number=w882) -> (unsigned 32bit integer=w903:u32)
            n294 = call-poly <vilib>:"DAQmx Read.vi"("task/channels in"=w894, "error in"=w897) -> ("task out"=w899:refnum<k21>, "data"=w888:u32, "error out"=w900:errorcluster)  [unwired: 11 in]
            n295 = Greater Or Equal?(x=w882, y=u32 1) -> (x >= y?=w879:bool)
            n296 = To Unsigned Long Integer(number=w888) -> (unsigned 32bit integer=w902:u32)
            n297 = call <vilib>:"DAQmx Clear Task.vi"("task in"=w899, "error in"=w900) -> ("error out"=w901:errorcluster)  [unwired: 13 in]
            n298 = Greater Or Equal?(x=w888, y=u32 1) -> (x >= y?=w886:bool)
            n299 = Select(t=u32 1 ("y"), s=w879, f=u32 0 ("y")) -> (s? t:f=w878:u32)
            n300 = call <vilib>:"DAQmx Clear Task.vi"("task in"=w898, "error in"=w901) -> ("error out"=w895:errorcluster)  [unwired: 13 in]
            n301 = Number To Decimal String(number=w878) -> (decimal integer string=w892:string)  [unwired: 1 in]
            n302 = Select(t=u32 1 ("y"), s=w886, f=u32 0 ("y")) -> (s? t:f=w883:u32)
            n303 = call-poly <vilib>:"DAQmx Write.vi"("task/channels in"=refnum<k21> "LaserChannel", "data"=FALSE) -> ()  [unwired: 11 in, 3 out]
            n304 = Number To Decimal String(number=w883) -> (decimal integer string=w891:string)  [unwired: 1 in]
            n305 = Concatenate Strings(w891, w892) -> (w889:string)
            n306 = case shown="\"11\"" w889 {
              tunnel: [w906 "Right" w913 "Left"] -> w890
              frame "00", Default {
                n307 = Random Number (0-1)() -> (number: 0 to 1=w907:dbl)
                n308 = Greater Or Equal?(x=w907, y=0.5) -> (x >= y?=w909:bool)
                n309 = Select(t="Left", s=w909, f="Right") -> (s? t:f=w906:string)
              }
              frame "10" {
              }
              frame "11" {
                n310 = Random Number (0-1)() -> (number: 0 to 1=w914:dbl)
                n311 = Greater Or Equal?(x=w914, y=0.5) -> (x >= y?=w916:bool)
                n312 = Select(t="Left", s=w916, f="Right") -> (s? t:f=w913:string)
              }
              frame "01" {
              }
            }
          }
          frame #5 {
            w922 = StateMachineStates_1."CleanUp"  # Next State
            n313 = local write "Stimulus"(TRUE ("Counts Taken")) -> ()
          }
        }
        n314 = local write "Photon #"(w831) -> ()
        n315 = local write "Counts 2"(w814) -> ()
        n316 = local write "Counts 1"(w816) -> ()
        n317 = local write "Observer \nchoice"(w813) -> ()
      }
      frame "WaitObserverResponse" {
        # "Accept user keyboard input and move to CleanUp phase when the spacebar is pressed."
        n318 = flat-sequence {
          tunnel: [w946] -> w942
          tunnel: [w948] -> w941
          tunnel: w942 -> [w948]
          tunnel: [w980] -> w939
          tunnel: [w974] -> w940
          tunnel: [w975] -> w938
          tunnel: w941 -> [w973]
          frame #0 {
            n319 = Get Date/Time In Seconds() -> (seconds since 1Jan1904=w946:timestamp)
            "Confidence" <- 0 ("Confidence")
          }
          frame #1 {
            n320 = while {
              stop <- w952 stop-if-true
              n321 = call "Query Keyboard.vi"("Stop?"=FALSE) -> ("element"=w950:T4)  [unwired: 9 in, 1 out]
              n322 = local read "Confidence"() -> (w955:i32)
              n323 = case shown="\"J\"..\"L\"" w950 {
                tunnel: ["Left" w961 "Right"] -> w951
                frame "D", "F", "S" {
                }
                frame Default {
                  n324 = local read "Observer \nchoice"() -> (w961:string)
                }
                frame "J".."L" {
                }
              }
              "Observer \nchoice" <- w951
              n325 = case shown="\"SPACE\"" w950 {
                tunnel: [FALSE TRUE] -> w954
                frame "0", Default {
                }
                frame "SPACE" {
                }
              }
              n326 = case shown="Default" w950 {
                tunnel: [0 1 2 3 3 2 1] -> w956
                frame Default {
                }
                frame "S" {
                }
                frame "D" {
                }
                frame "F" {
                }
                frame "J" {
                }
                frame "K" {
                }
                frame "L" {
                }
              }
              n327 = Greater Than 0?(x=w955) -> (x > 0?=w953:bool)
              n328 = And(x=w954, y=w953) -> (x .and. y?=w952:bool)
              n329 = Equal To 0?(x=w956) -> (x = 0?=w958:bool)
              n330 = And(x=w958, y=w953) -> (x .and. y?=w957:bool)
              n331 = Select(t=w955, s=w957, f=w956) -> (s? t:f=w959:i32)
              n332 = local write "Confidence"(w959) -> ()
            }
          }
          frame #2 {
            w980 = StateMachineStates_1."CleanUp"  # Next State
            n333 = Get Date/Time In Seconds() -> (seconds since 1Jan1904=w978:timestamp)
            n334 = local read "Confidence"() -> (w975:i32)
            n335 = Subtract(x=w978, y=w973) -> (x-y=w977:dbl)
            n336 = local read "Observer \nchoice"() -> (w974:string)
            n337 = Multiply(x=w977, y=1000.0) -> (x*y=→"Response \ntime (ms)":dbl)
            "Observer Responded" <- TRUE ("Boolean 3")
          }
        }
      }
      frame "CleanUp" {
        n338 = local read "Trial mode"() -> (w983:T1)
        n339 = local read "Subject #"() -> (w1006:string)
        n340 = case shown="True" "Audio" {
          tunnel: w1004 -> [_ w1076]
          tunnel: w1003 -> [_ w1075]
          frame False {
          }
          frame True {
            # "If audio is enabled, play sound for right or wrong answer."
            n341 = Equal?(x=w1076, y=w1075) -> (x = y?=w1077:bool)
            n342 = case shown="False" w1077 {
              frame False {
                n343 = call "Sound File to Sound Output.vi"("Volume"=100.0, "Number of Samples/Iteration"=10000, "Device ID"=u32 0, "File Path"=path "C:/Users/Lab/Dropbox/Vision software/chord_short.wav") -> ()
              }
              frame True {
                n344 = call "Sound File to Sound Output.vi"("Volume"=100.0, "Number of Samples/Iteration"=10000, "Device ID"=u32 0, "File Path"=path "C:/Users/Lab/Dropbox/Vision software/tada_short.wav") -> ()
              }
            }
          }
        }
        n345 = flat-sequence {
          tunnel: w1007 -> [w1031]
          tunnel: w1006 -> [w1028]
          tunnel: w1004 -> [w1024]
          tunnel: w1003 -> [w1023]
          tunnel: w1001 -> [w1022]
          tunnel: w1000 -> [w1020]
          tunnel: w999 -> [w1018]
          tunnel: w995 -> [w1013]
          tunnel: w985 -> [w1012]
          tunnel: [w1012] -> w984
          frame #0 {
            # "Write data from trial to file."
            n346 = Equal?(x=w1024, y=w1023) -> (x = y?=w1038:bool)
            n347 = local read "Photon #"() -> (w1015:i32)
            n348 = local read "Photon time (ms)"() -> (w1011:dbl)
            n349 = local read "LED Voltage"() -> (w1016:dbl)
            n350 = local read "Response \ntime (ms)"() -> (w1027:dbl)
            n351 = Select(t=1.0, s=w1038, f=0.0) -> (s? t:f=w1035:dbl)
            n352 = To Long Integer(number=w1027) -> (32bit integer=w1030:i32)
            n353 = To Long Integer(number=w1035) -> (32bit integer=w1034:i32)
            n354 = Number To Engineering String(2:i16 2 ("width (-)"), 4:w1016) -> (0:w1026:string)  [unwired: 2 in]
            n355 = Number To Decimal String(number=w1013) -> (decimal integer string=w1017:string)  [unwired: 1 in]
            n356 = Number To Decimal String(number=w1015) -> (decimal integer string=w1014:string)  [unwired: 1 in]
            n357 = Number To Decimal String(number=w1030) -> (decimal integer string=w1029:string)  [unwired: 1 in]
            n358 = Number To Decimal String(number=w1034) -> (decimal integer string=w1033:string)  [unwired: 1 in]
            n359 = Number To Decimal String(number=w1022) -> (decimal integer string=w1021:string)  [unwired: 1 in]
            n360 = Number To Decimal String(number=w1020) -> (decimal integer string=w1019:string)  [unwired: 1 in]
            n361 = Number To Decimal String(number=w1031) -> (decimal integer string=w1032:string)  [unwired: 1 in]
            n362 = Number To Decimal String(number=w1011, width (-)=i16 5) -> (decimal integer string=w1010:string)
            n363 = Build Array(w1028, w1017, w1024, w1026, w1014, w1023, w1029, w1032, w1033, w1021, w1019, w1010) -> (w1039:string[])
            n364 = call "Write Data.vi"("Trial Results"=w1039, "base path"=w1018) -> ()  [unwired: 10 in]
          }
        }
        n365 = Array Size(array=w997) -> (size(s)=w996:i32)
        n366 = Equal?(x=w983, y=T1."Mixed LED") -> (x = y?=w981:bool)
        n367 = flat-sequence {
          tunnel: w984 -> [w1050]
          tunnel: [w1050] -> w990
          tunnel: w989 -> [w1043]
          tunnel: [w1044] -> w988
          tunnel: [w1041] -> w987
          tunnel: w981 -> [w1040]
          tunnel: [w1054] -> w991
          tunnel: w990 -> [w1054]
          frame #0 {
            # "Increment blocked trial # if not in manual mode or\nan LED trial (mixed mode)."
            n368 = feedback #7(0) -> (w1045:i32)
            n369 = local read "Bright trial\nrequested"() -> (w1041:bool)
            n370 = Compound Arithmetic op=OR(w1041, w1043, w1040) -> (w1042:bool)
            n371 = Select(t=0, s=w1042, f=1) -> (s? t:f=w1048:i32)
            n372 = Add(x=w1045, y=w1048) -> (x+y=w1044:i32)
            "Blocked trial #" <- w1044
            n373 = feedback-in #7(w1044) -> ()
          }
          frame #1 {
            w1053 = FALSE ("LC")
            # "Reset indicators"
            n374 = local write "Photon #"(0 ("Photon #")) -> ()
            n375 = local write "Stimulus"(w1053) -> ()
            n376 = local write "Observer Ready"(w1053) -> ()
            n377 = local write "Location Set"(w1053) -> ()
            n378 = local write "Waiting"(w1053) -> ()
            n379 = local write "Bright trial\nrequested"(w1053) -> ()
            n380 = local write "LED Voltage"(0.0 ("LED Voltage")) -> ()
          }
        }
        n381 = Equal?(x=w996, y=w988) -> (x = y?=w994:bool)
        n382 = Not(x=w989) -> (.not. x?=w998:bool)
        n383 = And(x=w998, y=w994) -> (x .and. y?=w993:bool)
        n384 = case shown="False" w993 {
          tunnel: [w1057 w1069] -> w1008
          tunnel: w989 -> [w1055 _]
          tunnel: [w1055 w1068] -> w992
          frame False {
            # "Display a message and\nswitch to manual mode\nif end of blocked trials\nis reached."
            n385 = case shown="True" "Self-paced" {
              tunnel: [w1059 w1064] -> w1057
              frame False {
                n386 = call "Display Message to User"() -> ("OK"=w1058:bool)  [unwired: 10 in, 1 out]
                n387 = case shown="True" w1058 {
                  tunnel: [w1060 w1062] -> w1059
                  frame False {
                    w1060 = StateMachineStates_1."CleanUp"  # Next State
                  }
                  frame True {
                    w1062 = StateMachineStates_1."WaitResearcher"  # Next State
                    n388 = local write "Observer Responded"(FALSE ("Observer Responded")) -> ()
                  }
                }
              }
              frame True {
                # "Skip \"WaitingResearcher\" mode if trials are self-paced."
                n389 = local write "Observer Responded"(FALSE ("Observer Responded")) -> ()
                n390 = local read "L/R control method"() -> (w1063:enum16{"Liquid crystal", "Motorized waveplate"})
                n391 = case shown="\"Motorized waveplate\"" w1063 {
                  tunnel: [w1066 w1067] -> w1064
                  frame "Liquid crystal", Default {
                    w1066 = StateMachineStates_1."SetLC"  # Next State
                  }
                  frame "Motorized waveplate" {
                    w1067 = StateMachineStates_1."SetWP"  # Next State
                  }
                }
              }
            }
          }
          frame True {
            w1068 = TRUE ("Manual")
            n392 = local write "Self-paced"(FALSE ("Self-paced")) -> ()
            n393 = local write "Manual"(w1068) -> ()
            n394 = call "Display Message to User2"() -> ("OK"=w1070:bool)  [unwired: 10 in, 1 out]
            n395 = case shown="True" w1070 {
              tunnel: [w1072 w1074] -> w1069
              frame False {
                w1072 = StateMachineStates_1."CleanUp"  # Next State
              }
              frame True {
                w1074 = StateMachineStates_1."WaitResearcher"  # Next State
                n396 = local write "Observer Responded"(FALSE ("Observer Responded")) -> ()
              }
            }
          }
        }
      }
      frame "Stop" {
        n397 = flat-sequence {
          tunnel: w1090 -> [w1104]
          tunnel: w1089 -> [w1103]
          tunnel: [w1105] -> w1088
          tunnel: w1088 -> [w1107]
          tunnel: [w1107] -> w1087
          tunnel: [w1109] -> w1091
          tunnel: w1087 -> [w1109]
          tunnel: [StateMachineStates_1."Stop" ("Next State")] -> w1086
          frame #0 {
            # "Close waveplate session."
            n398 = call "close.vi"("error in"=w1104, "VISA Handle in"=w1103) -> ("error out"=w1105:errorcluster)  [unwired: 3 in]
          }
          frame #1 {
            w1106 = FALSE ("LC")
            # "Reset indicator lights."
            n399 = local write "Observer Ready"(w1106) -> ()
            n400 = local write "Stimulus"(w1106) -> ()
            n401 = local write "Location Set"(w1106) -> ()
            n402 = local write "Observer Responded"(w1106) -> ()
            n403 = local write "Waiting"(w1106) -> ()
          }
          frame #2 {
          }
        }
      }
    }
  }
